vi "AlliGator Phasor Plot Actions.vi"(0 "AlliGator Q Elements in":T6[](array[typedef]), 1 "VI in":refnum<vi>, 2 "Script in":bool, 5 "data value reference in":refnum<data-value>, 7 "AlliGator Q Event in":T7=enum."GUI:Idle", 9 "Data":variant, 11 "error in (no error)":errorcluster, 12 "AlliGator Ctrl Refnums":T8) -> (3 "Script out":bool, 4 "AlliGator Q Elements out":T6[](array[typedef]), 6 "Data Value Reference out":refnum<data-value>, 10 "[Notebook Message]":T1[](array[typedef]) {"Message Style"."Font Size" min=6.0 step=1.0}, 15 "error out":errorcluster)   [LabVIEW 2021, in "AlliGator Action Engine.lvlib"]
doc: "Processes AlliGator phasor plot-related actions."
uses:
  AlliGator Action Engine.lvlib
  Internal Variables/AlliGator Internal Variables v2.ctl
  <vilib>/vision/Image Controls.llb/IMAQ Image.ctl
  Internal Variables/AlliGator Gate Image Set.ctl
  Files/AlliGator FLI Dataset Type.ctl
  Files/AlliGator Data Series Type.ctl
  Dual-Channel Datasets/AlliGator Dataset Channel.ctl
  Settings/AlliGator Gate Arithmetic.ctl
  Source Image/AlliGator Displayed Image.ctl
  Image/Named ROI Description.ctl
  Phasor Graph/AlliGator Decay Metadata v3.ctl
  Decay Analysis/Decay Preprocessing/AlliGator Decay Background Subtraction Info.ctl
  Decay Analysis/Decay Preprocessing/AlliGator Baseline Subtraction Method.ctl
  Graphs/XY Graph/XY Graph Plot Shift Parameters.ctl
  Graphs/XY Graph/XY Graph Plot Shift Method.ctl
  Decay Analysis/Decay Preprocessing/AlliGator Decay Extrapolation Parameters.ctl
  Phasor/Calibration Phasor (m, phi).ctl
  Phasor/Phasor Reference Series.ctl
  Phasor/Phasor Calibration Map v2.ctl
  Phasor/Phasor (g, s).ctl
  Phasor Graph/AlliGator Raw Phasor Plot Data v5.ctl
  Phasor/Phasor Standard Deviation Options.ctl
  Phasor Plot/AlliGator Phasor Multi-Harmonic Data.ctl
  Phasor/Phasor Harmonic Data.ctl
  Decay Fit Parameter Map/AlliGator Decay Fit Options & Parameters v4.ctl
  Fits/IRF(X)PSED/Decay Fit Options v4.ctl
  Fits/Decay Convolution/Decay Model.ctl
  Fits/Residual Type.ctl
  Fits/IRF(X)PSED/Fit Weights Type v2.ctl
  Fits/Non-linear Fitting Method v2.ctl
  Fits/Fit Calculation Method.ctl
  Fits/Non-linear Fitting Algorithm.ctl
  Decay Analysis/Decay Fit/AlliGator Decay Fit Parameter Constraints 2.ctl
  Fits/IRF(X)PSED/Decay Fit Parameters In List.ctl
  Fits/IRF(X)PSED/MLE Baseline Offset Type.ctl
  Decay Analysis/Decay Preprocessing/AlliGator Decay Preprocessing Parameters.ctl
  Fits/IRF(X)PSED/Decay Fit Parameters & Derived Quantities List v2.ctl
  Fits/IRF(X)PSED/Decay Fit Result Constraint.ctl
  Decay Fit Parameter Map/AlliGator Parameter Maps Data.ctl
  AlliGator Q Event.ctl
  GUI/AlliGator Ctrl Refnums.ctl
  GUI/AlliGator Other Ctrl Refnums.ctl
  GUI/AlliGator State Indicator.ctl
  GUI/AlliGator Main Window Tabs.ctl
  GUI/AlliGator Phasor Plot Ctrl Refnums.ctl
  GUI/AlliGator Phasor Graph Ctrl Refnums.ctl
  Phasor/Phasor Calibration Type.ctl
  GUI/AlliGator Dataset Ctrl Refnums.ctl
  GUI/AlliGator Registered Events Ctrl Refnums.ctl
  GUI/AlliGator Image Histogram Control Refnums.ctl
  Histograms/Linear Histogram Options.ctl
  Histograms/Histogram Bin Option.ctl
  Histograms/Histogram Bin Position.ctl
  Decay Fit Parameter Map/AlliGator Decay Fit Map Control Refnums.ctl
  Parameter Map/AlliGator Parameter Map Control Refnums.ctl
  AlliGator Q Element.ctl
  Notebook/Notebook Message Object.ctl
  Rich Text Box/Text Formatting.ctl
  Rich Text Box/Text Colors.ctl
  Rich Text Box/Text Style.ctl
  Rich Text Box/Text Alignment.ctl
  Rich Text Box/Text Format List.ctl
  Globals, Variables, Constants/AlliGator Variables List.ctl
  GUI/AlliGator Image Display Type.ctl
  Palette/Image Palette Information.ctl
  Image/Image Display Palette Type.ctl
  Alligator Elements Order in Action Stack.ctl
  Image/Image Control ROI Description.ctl
  Settings/AlliGator Settings List.ctl
  ROIs/AlliGator ROI Manager Actions.ctl
  Utilities/Read-Write.ctl
  793a9f64-fd61-4161-b52c-76edb5dbf837.vi
  Variant/Variant to Data/Variant to Boolean.vi
  Variant/Variant to Data/Variant to [String].vi
  AlliGator Add Single Action to Stack.vi
  Variant/Variant to Data/Variant to String.vi
  Variant/Variant to Data/Variant to IMAQ Image.vi
  AlliGator Add Action Array to Stack.vi
  ROIs/AlliGator Phasor Plot Image ROI Storage [SGL] v3.vi
  Variant/Variant to Data/Variant to Data.lvlib
  GUI/GUI.lvlib
  Phasor Plot/AlliGator Phasor Plot.lvlib
  Phasor Ratio/AlliGator Phasor Ratio.lvlib
  Phasor Plot Color Map/AlliGator Phasor Plot Color Map.lvlib
  Image/Image.lvlib
  Source Image/AlliGator Source Image.lvlib
  Files/AlliGator Files.lvlib
  Internal Variables/AlliGator Internal Variables.lvlib
  Files/Files.lvlib
  GUI/AlliGator GUI.lvlib
  Globals, Variables, Constants/AlliGator Globals, Variables & Constants.lvlib
  Palette/Palette.lvlib
  ROIs/AlliGator ROIs.lvlib
  Settings/AlliGator Settings.lvlib
  Utilities/Utilities.lvlib
  Sound/Sound.lvlib
  <vilib>/Utility/miscctls.llb/LVPoint32TypeDef.ctl
  Image/Image Control Refnum.ctl
  Image/Image Display Mouse Click Event Data.ctl
  Time/Time.lvlib
  Phasor/Phasor.lvlib
  Notebook/Notebook.lvlib
  Decay Analysis/Decay Preprocessing/AlliGator Decay Preprocessing.lvlib
  Graphs/XY Graph/XY Graph Add-Ons.lvlib
  Phasor Graph/AlliGator Phasor Graph.lvlib
  Fits/Fits.lvlib
  Decay Analysis/Decay Fit/AlliGator Decay Fit.lvlib
  Decay Fit Parameter Map/AlliGator Decay Fit Parameter Map.lvlib
  Rich Text Box/Rich Text Box.lvlib
  Dual-Channel Datasets/AlliGator Dual-Channel Datasets.lvlib
  Histograms/Histogram Window.lvlib
  Parameter Map/AlliGator Parameter Map.lvlib
panel:
  # "see the AlliGator License on the block diagram (Ctrl+E or Window:Show Block Diagram)"
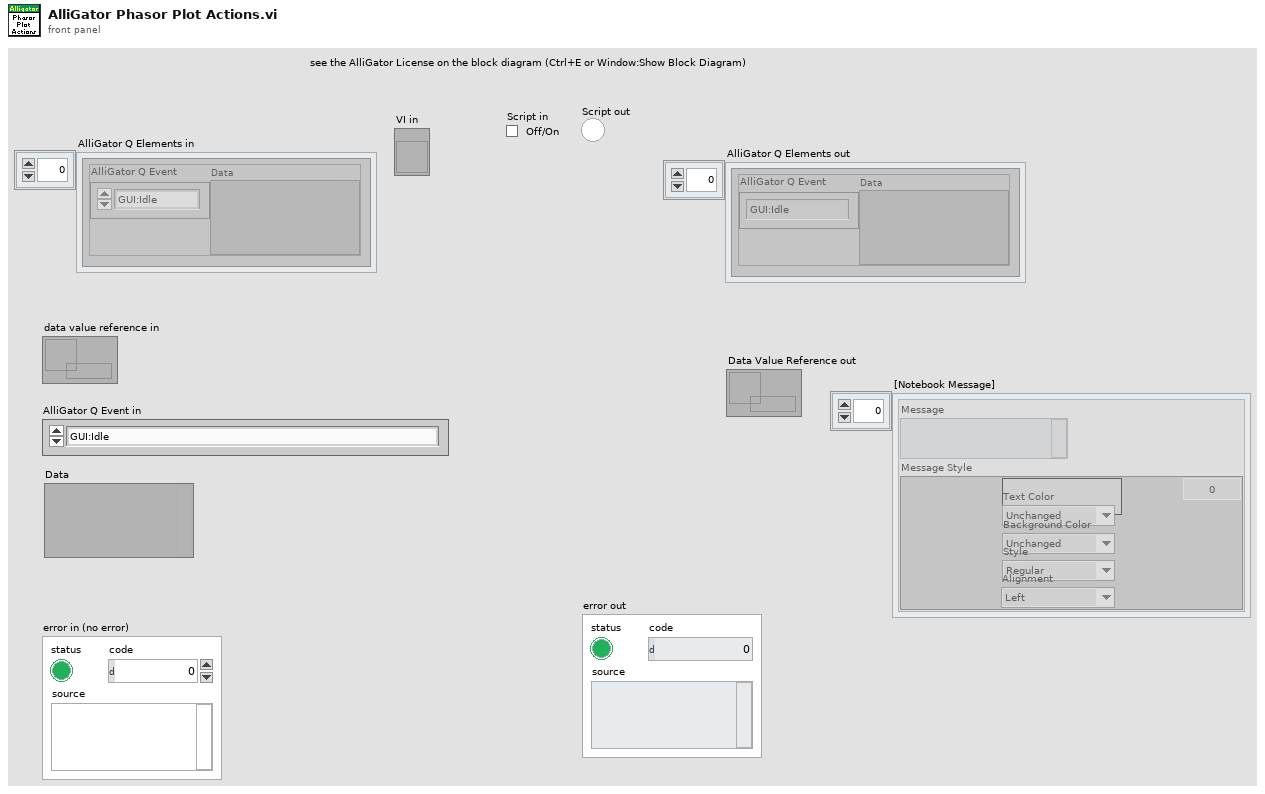
[diagram p1: front panel]
types:
  T1 = typedef "Notebook.lvlib/Notebook Message Object.ctl" = cluster{"Message":string, "Message Style":T2}
  T2 = typedef "Rich Text Box.lvlib/Text Formatting.ctl" = cluster{"Font":string, "Text Color":T3, "Background Color":T3, "Style":T4, "Font Size":dbl, "Alignment":T5}
  T3 = typedef "Rich Text Box.lvlib/Text Colors.ctl" = enum16{"Unchanged", "Black", "Blue", "Cyan", "Maroon", "Gray", "Violet", "Green", "Light Green", "Orange", "Yellow", "Magenta", "Red", "White"}
  T4 = typedef "Rich Text Box.lvlib/Text Style.ctl" = enum16{"Regular", "Bold", "Italic", "Underline", "Strikeout"}
  T5 = typedef "Rich Text Box.lvlib/Text Alignment.ctl" = enum16{"Left", "Right", "Center"}
  T6 = typedef "AlliGator Action Engine.lvlib/AlliGator Q Element.ctl" = cluster{"AlliGator Q Event":T7, "Data":variant}
  T7 = typedef "AlliGator Action Engine.lvlib/AlliGator Q Event.ctl" = enum16{"---- Files ----", "Files:Set Batch Export Files To Save", "Files:Set Dataset Loading & Pre-processing Options", "Files:Check #Frames in Dataset", "Files:Increment Frame Index", "Files:Open Mask Image", "Files:Open White Light Image", "Files:Open Single Dataset", "Files:New Folder of Folders Selected", "Files:Load File (all Types)_Scriptable", "Files:Move Flattened Series to Folders Series", "Files:Select Folder", "Files:Load FLI Dataset", "Files:Load Swiss SPAD 1 Dataset", "Files:Load Swiss SPAD 2 Dataset", "Files:Load .sdt FLI Dataset", "Files:Load .ptu FLI Dataset", "Files:Load .bin FLI Dataset", "Files:Load Single Gate Image Folder", "Files:Load I/m/phi Dataset (deprecated)", "Files:Load Single Image", "Files:Subtract Background File", "Files:Export FLI Dataset", "Files:Load HDF5 FLI Dataset", "Files:Set Destination File Path", "Files:Save Mask Image", "Files:Batch Conversion", "Files:New Folder Selected", "Files:Close FLI Dataset", "Files:Close FLI Dataset Series", "Files:Close White Light Image", "Files:Close Mask Image", "---- FLI Dataset ----", "FLI Dataset:Channel Arithmetic", "FLI Dataset:Export Average Lifetime Map as ASCII", "FLI Dataset:Export User-Defined Quantity Map as ASCII", "FLI Dataset:Python Function FLI Dataset Event", "FLI Dataset:ROI Analysis", "FLI Dataset:Tilted Logistic Square Gated IRF Characteristics Map", "FLI Dataset:Logistic Square Gated IRF Characteristics Map", "FLI Dataset:Square Gated IRF Characteristics Map", "FLI Dataset:Multi-ROI Single-Pixel Phasor Analysis", "FLI Dataset:Multi-ROI Single-Pixel NLSF Analysis", "FLI Dataset:All ROIs IRF Extraction", "FLI Dataset:All ROIs Decay Fit Non-Interactive (Fast + Individual IRF)", "FLI Dataset:All ROIs Phasor Analysis", "FLI Dataset:All ROIs Decay Fit", "FLI Dataset:Fluorescence Decay Statistics", "FLI Dataset:Update Decay Statistics Graph", "FLI Dataset:Get Decay from ROI", "FLI Dataset:All ROIs Average Lifetimes", "FLI Dataset:Save/Load Local IRFs", "FLI Dataset:Clear Local IRFs", "FLI Dataset:Phasor Calibration Maps (# Gates Series) Script", "FLI Dataset:Calibrated Phasor Map Series", "---- FLI Dataset Series ----", "FLI Dataset Series:Sum All Datasets in Series", "FLI Dataset Series:Add Dataset to Accumulated Dataset", "FLI Dataset Series:Display Accumulated Dataset", "FLI Dataset Series:Clear Dataset Series Sum", "FLI Dataset Series:Time-Series Analysis (NLSF)", "FLI Dataset Series:Time-Series Analysis (Phasor)", "---- Image ----", "Image:Update Image Profile Plots", "Image:Image Histogram Cursor Move", "Image:Image Histogram", "Image:Image Contrast", "Image:Set Image Histogram Cursor Move Flag", "Image:Clear Image Overlay", "Image:Use ROI as Search Area", "Image:Set ROI Diameter", "Image:Save Image Data as TIFF", "Image:Save Displayed Image with Overlay", "Image:Save Image Overlay Only", "Image:Save Image as Hot Pixel Mask", "Image:Change Source Image Color Palette", "Image:Copy Image to Clipboard", "Image:Source Image ROI Selection", "Image:Delete All ROIs", "Image:Delete All Unselected ROIs", "Image:Delete ROI", "Image:Merge All ROIs", "Image:Store ROI", "Image:Source Image ROI Storage", "Image:Export ROI Description to Notebook", "Image:Save ROI", "Image:Load ROI", "Image:Paste ROI Definition", "Image:Clear ROI", "Image:Identify ROIs in Mask Image", "Image:Create Complementary ROI", "Image:Create Contour ROI", "Image:Create ROI(s) from Pixels with Peak above Min_Scriptable", "Image:Create ROI(s) from Pixels with Intensity above Min_Scriptable", "Image:Compute ROI Statistics", "Image:Delete ROI(s) based on ROI Characteristics", "Image:Create ROI Grid", "Image:ROI to Individual Pixel ROIs", "Image:Python Function Source Image Event", "Image:Show Phasor Calibration Map ROI Centers", "Image:Convert ROI to Mask Image", "Image:Mouse Move", "Image:Mouse Up", "Image:Set Source Image Mouse Move Flag", "Image:Add Scale Bar Overlay", "Image:Delete Existing ROIs Option", "Image:Overlay ROI Median", "Image:Check Current ROI", "Image:Update True Pixel Value", "---- Decay ----", "Decay:Clear IRF/Reference Plot", "Decay:Add Decay to Graph", "Decay:Smoothen Plot", "Decay:Smoothen Plot Tail", "Decay:Average Selected Plots", "Decay:Extract IRF", "Decay:Optimal IRF Extraction", "Decay:Threshold IRF", "Decay:Fit to Model IRF", "Decay:Fit IRF to Square Gate", "Decay:Fit IRF to Logistic Square Gate", "Decay:Fit IRF to Tilted Logistic Square Gate", "Decay:Create Bounding Cursors Set", "Decay:Export Bounding Cursors Definition to Notebook", "Decay:Denoise Plot", "Decay:Compute Cumulative Function", "Decay:Use as Reference Decay", "Decay:Show Reference Decay/IRF", "Decay:Extrapolate Decay", "Decay:Create Head & Tail Bounding Cursors", "Decay:Store Cursor-defined Head & Tail Fractions", "Decay:Rebin Plot", "Decay:1-Normalize Decay", "Decay:[0-1]-Normalize Plot", "Decay:Straighten Decay", "Decay:Shift Decay", "Decay:Fold Decay", "Decay:Fit Decay", "Decay:Global Fit of Selected Decays", "Decay:Post Global Fit Script", "Decay:Add Global Fit Parameters to Graph", "Decay:Add Decay Parameter(s) to Plot (Graph)", "Decay:Export Decay to Phasor Graph", "Decay:Compute Average Lifetime", "Decay:Plot Convolution", "Decay:Graph Tip Strip Update", "---- Decay Statistics ----", "Decay Statistics:Tip Strip Update", "---- Intensity Time Trace ----", "Intensity Time Trace:Use File Timestamp", "Intensity Time Trace:Load Intensity Corrections File", "Intensity Time Trace:Clear Intensity Corrections File", "Intensity Time Trace:Tip Strip Update", "---- Phasor Plot ----", "Phasor Plot:Build Phasor Plot", "Phasor Plot:Change Phasor Plot Color Palette", "Phasor Plot:Adjust Phasor Plot Display Range", "Phasor Plot:Highlight Image ROI in Phasor Plot", "Phasor Plot:Save Phasor Plot Image with Overlay", "Phasor Plot:Export Complex Phasor Map", "Phasor Plot:Export Phasor Ratio Map", "Phasor Plot:Export Average Lifetime Map", "Phasor Plot:Compute Phase Lifetime Histogram", "Phasor Plot:Compute Phasor Ratio Histogram", "Phasor Plot:Compute Phase Lifetime vs Intensity Scatter Plot", "Phasor Plot:Weber 2-Component Decomposition", "Phasor Plot:Update Phasor Color Map Vertices", "Phasor Plot:Clear Phasor Overlay", "Phasor Plot:Use Segment Extremities as References", "Phasor Plot:Use UC/Segment Intersections as References", "Phasor Plot:Use UC/Principal Axis Intersections as References", "Phasor Plot:Use UC/Linear Fit Intersections as References", "Phasor Plot:Update Phasor Plot Reference", "Phasor Plot:Show Local Phasor Info in Phasor Plot", "Phasor Plot:Update Phasor Plot State", "Phasor Plot:Phasor Plot ROI Storage", "Phasor Plot:Phasor Plot ROI Selection", "Phasor Plot:Python Function Phasor Plot Event", "Phasor Plot:Overlay Phasor ROI, Ratio or Map in Source Image", "Phasor Plot:Compute Decay of Selected Phasors", "Phasor Plot:Phasor at Image Pixel", "Phasor Plot:Mouse Move", "Phasor Plot:Mouse Up", "Phasor Plot:Display Range Mouse Move", "Phasor Plot:Set Mouse Move Flag", "Phasor Plot:Update True Phasor Plot Value", "---- Phasor Graph ----", "Phasor Graph:Get Phasor Value", "Phasor Graph:Create New Phasor Plot Dialog", "Phasor Graph:Update Last Phasor Value", "Phasor Graph:Update Phasor (m, phi)", "Phasor Graph:Remove Single Phasor from Plot", "Phasor Graph:Add Single Phasor to Plot", "Phasor Graph:Remove Phasor Plot", "Phasor Graph:Remove Selected Phasor Plots", "Phasor Graph:Clear Phasor Data", "Phasor Graph:Clear Phasor Graph", "Phasor Graph:Cursor Move", "Phasor Graph:Draw Cursor Connecting Line", "Phasor Graph:Clear Cursor Connecting Line", "Phasor Graph:Find UC Intersection", "Phasor Graph:Use UC/Cursor-Defined Line Intersections", "Phasor Graph:Use Selected Plots Fitted Line/UC Intersections", "Phasor Graph:Use Selected Plots Principal Axis/UC Intersections", "Phasor Graph:Show Single Phasor", "Phasor Graph:Save Single Phasor Plot", "Phasor Graph:Save All Phasor Plots", "Phasor Graph:Load Phasor Plot(s)", "Phasor Graph:Phasor Multiplication", "Phasor Graph:Compute Average Phasor", "Phasor Graph:Compute Multiple Average Phasors (Selected Plots)", "Phasor Graph:Export Single Phasor Plot Phase Lifetimes", "Phasor Graph:Parameter 2 vs Parameter 1 Scatter Plot", "Phasor Graph:Use Cursor n Location", "Phasor Graph:Set Reference n to Current Phase Lifetime Value", "Phasor Graph:Set Reference n to Lifetime Value", "Phasor Graph:Set Cursor n Location", "Phasor Graph:Save Phasor Graph Image", "Phasor Graph:Update SEPL Plot", "Phasor Graph:Export Single Phasor Plot Data", "Phasor Graph:Export Selected Phasor Plots Data", "Phasor Graph:Python Function Phasor Graph Event", "Phasor Graph:Tip Strip Update", "---- Calibration ----", "Calibration:Set Calibration Type", "Calibration:Load/Save Phasor Calibration", "Calibration:Load/Save Phasor Calibration Series", "Calibration:Load/Save Phasor Calibration Map", "Calibration:Use as Calibration", "Calibration:Compute Optimal Calibration from Phasor References", "Calibration:Clear Phasor Calibration", "Calibration:Single Phasor Calibration Information", "Calibration:Use as Calibration Series", "Calibration:Use as Calibration Map", "Calibration:Clear Calibration Series", "Calibration:Phasor Calibration Series Information", "Calibration:Clear Calibration Map", "Calibration:Phasor Calibration Map Information", "Calibration:Apply Phasor Calibration", "Calibration:Update Single Plot Calibration", "Calibration:Update Multiple Plots Calibration", "Calibration:Clear Single Plot Calibration", "Calibration:Clear All Plots Calibrations", "Calibration:Clear Plot(s) Calibration(s)?", "---- Phasor Ratio ----", "Phasor Ratio:Clear Reference n", "Phasor Ratio:Toggle Selected Plot(s)  Lock to Reference 1", "Phasor Ratio:Use as Reference n", "Phasor Ratio:Send Reference n to Notebook", "Phasor Ratio:Toggle Selected Plot(s)  Lock to Reference 2", "Phasor Ratio:Compute Phasor Ratio at Mouse Location", "Phasor Ratio:Compute Phasor Plot's Average Phasor Ratio", "Phasor Ratio:Compute Time-Series Phasor Ratios", "Phasor Ratio:Fit Line to Phasor Ratio Plot", "Phasor Ratio:Save References", "Phasor Ratio:Load References", "Phasor Ratio:Update Phasor Reference 1", "Phasor Ratio:Update Phasor Reference 2", "Phasor Ratio:Move Cursor n to Reference n", "Phasor Ratio:Use as Phasor Reference 1 Lifetime", "Phasor Ratio:Use as Phasor Reference 2 Lifetime", "Phasor Ratio:Export Phasor Ratio Map as ASCII", "Phasor Ratio:Tip Strip Update", "---- Lifetime & Other Parameters Graph ----", "Lifetime:Compute Sliced Mean, SDV and CV Plots", "Lifetime:Plot Decay Shifts", "Lifetime:Plot Histogram", "---- Decay Fit Parameter Map ----", "Decay Fit Parameter Map:Export ROI NLSF Data as ASCII", "Decay Fit Parameter Map:Set Decay Fit Parameter Map Selection", "Decay Fit Parameter Map:Build Decay Fit Parameter Map", "Decay Fit Parameter Map:Change Decay Fit Parameter Map Color Palette", "Decay Fit Parameter Map:Export Decay Fit Parameter Map Data as ASCII", "Decay Fit Parameter Map:Export All Decay Fit Parameter Maps Data as ASCII", "Decay Fit Parameter Map:Selected Parameter Scatterplot", "Decay Fit Parameter Map:Parameter 2 vs Parameter 1 Scatterplot", "Decay Fit Parameter Map:Save Decay Fit Parameter Map Image", "Decay Fit Parameter Map:Save-Load IRFs & Fit Data", "Decay Fit Parameter Map:Update Local Decay Plots", "Decay Fit Parameter Map:Python Function Decay Fit Parameters Map Event", "Decay Fit Parameter Map:Overlay Decay Fit Parameter Map in Source Image", "Decay Fit Parameter Map:Selected Parameter vs Intensity Scatterplot", "Decay Fit Parameter Map:Mouse Up", "Decay Fit Parameter Map:Mouse Move", "Decay Fit Parameter Map:Display Range Mouse Move", "Decay Fit Parameter Map:Change Map Resolution", "Decay Fit Parameter Map:Variance Significance Maps", "Decay Fit Parameter Map:Fit Result Constraints Window", "---- Parameter Map ----", "Parameter Map:Export ROI Parameters Data as ASCII", "Parameter Map:Add Parameter Map Set", "Parameter Map:Delete Parameter Map Set", "Parameter Map:Update Parameter List", "Parameter Map:Build Parameter Map", "Parameter Map:Change Parameter Map Color Palette", "Parameter Map:Export Parameter Map Data as ASCII", "Parameter Map:Export All Parameter Maps Data as ASCII", "Parameter Map:Selected Parameter Scatterplot", "Parameter Map:Parameter 2 vs Parameter 1 Scatterplot", "Parameter Map:Selected Parameter vs Intensity Scatterplot", "Parameter Map:Save Parameter Map Image", "Parameter Map:Save-Load IRFs & Parameter Maps (TODO)", "Parameter Map:Set Parameter Map Selection", "Parameter Map:Python Function Parameter Map Event", "Parameter Map:Overlay Parameter Map in Source Image", "Parameter Map:Update Local Decay Plots", "Parameter Map:Mouse Up", "Parameter Map:Mouse Move", "Parameter Map:Display Range Mouse Move", "---- Generic Graph ----", "Generic Graph:Generic XY Graph Event", "Generic Graph:Python Function XY Graph Event", "Generic Graph:New Plot", "Generic Graph:Save Plot", "Generic Graph:XY Plot Histogram", "Generic Graph:Set XY Graph Plot Name", "Generic Graph:Set Last Cursor Style", "Generic Graph:Tip Strip Update", "---- GUI ----", "GUI:Start Script", "GUI:Type of Displayed Image Changed", "GUI:Gate Image Slide Changed", "GUI:Show Busy Icon", "GUI:Show Busy Icon & Abort Button", "GUI:Hide Busy Icon", "GUI:Hide Busy Icon & Abort Button", "GUI:Abort", "GUI:End Script", "GUI:Start Timing", "GUI:End Timing", "GUI:Set State Indicator", "GUI:Send Parameters JSON Strings to Clipboard", "GUI:Set Gate Step", "GUI:Idle", "GUI:Initialization", "GUI:Quit", "GUI:Increment Dataset Index", "GUI:Set Dataset Index to -1", "GUI:Time Series Slider Moved", "GUI:Time Series Slider Changed", "GUI:Toggle Playback or Loop", "GUI:Playback Script", "GUI:Set Phasor Frequency", "GUI:Open Window", "GUI:Start Test Script", "GUI:End Test Script", "GUI:Set Verbose Mode", "GUI:Set Verbose Settings Mode", "DEBUG"}
  T8 = typedef "AlliGator GUI.lvlib/AlliGator Ctrl Refnums.ctl" = cluster{"Other AlliGator Ctrl Refnums":T9, "Phasor Plot Ctrl Refnums":T10, "Phasor Graph Ctrl Refnums":T11, "Dataset Control Refnums":T12, "Registered Events Ctrl Refnums":T13, "Image Histogram Ctrl Refnums":T14, "Decay Fit Map Ctrl Refnums":T15, "Parameter Map Ctrl Refnums":T16}
  T9 = typedef "AlliGator GUI.lvlib/AlliGator Other Ctrl Refnums.ctl" = cluster{"State Indicators":refnum<vi>, " Progress Bar":refnum<vi>, "Decay Graph Active":refnum<vi>, "Decay Statistics Bin":refnum<vi>, "Time Step":refnum<vi>, "Use File Timestamp":refnum<vi>, "Tab Control":refnum<vi>, "CPU":refnum<vi>, "Abort Fit":refnum<vi>, "Dataset File/Folder Path":refnum<vi>, "Abort ROI Creation":refnum<vi>, "Event LED":refnum<vi>, "Dataset File/Folder Path 2":refnum<vi>, "Dataset File/Folder Path 3":refnum<vi>, "Dataset File/Folder Path 4":refnum<vi>, "Dataset File/Folder Path 5":refnum<vi>, "Dataset File/Folder Path 6":refnum<vi>, "Dataset File/Folder Path 7":refnum<vi>, "Dataset File/Folder Path 8":refnum<vi>, "Dataset File/Folder Path 9":refnum<vi>, "Dataset File/Folder Path 10":refnum<vi>, "Dataset File/Folder Path 11":refnum<vi>}
  T10 = typedef "AlliGator GUI.lvlib/AlliGator Phasor Plot Ctrl Refnums.ctl" = cluster{"Phasor Ratio":refnum<vi>, "Modulus Lifetime":refnum<vi>, "Phasor at cursor (m, phi)":refnum<vi>, "Phase Lifetime":refnum<vi>, "Phasor at cursor (g, s)":refnum<vi>, "Phasor Plor Average Lifetime":refnum<vi>, "Phasor Plot Active":refnum<vi>, "Save Phasor Plot":refnum<vi>, "Image Overlay Color":refnum<vi>, "Phasor Plot Color Scale":refnum<vi>, "Reference 1 Button":refnum<vi>, "Reference 2 Button":refnum<vi>, "True Phasor Plot Value":refnum<vi>}
  T11 = typedef "AlliGator GUI.lvlib/AlliGator Phasor Graph Ctrl Refnums.ctl" = cluster{"Phasor Ratio":refnum<vi>, "Modulus Lifetime":refnum<vi>, "Phasor at cursor (m, phi)":refnum<vi>, "Phase Lifetime":refnum<vi>, "Phasor at cursor (g, s)":refnum<vi>, "Phasor Graph Average Lifetime":refnum<vi>, "Phasor Graph Active":refnum<vi>, "Save Phasor Graph":refnum<vi>, "Phasor Frame Slide":refnum<vi>, "Single Step Phasor":refnum<vi>, "Calibration Type":refnum<vi>, "Show Line":refnum<vi>, "Phase Lifetime 1":refnum<vi>, "Phase Lifetime 2":refnum<vi>, "Phasor Graph Frequency":refnum<vi>, "Phasor Reference 1 Control":refnum<vi>, "Phasor Reference 2 Control":refnum<vi>, "Calibration Lifetime":refnum<vi>, "Phase Lifetime SDV":refnum<vi>, "Average Lifetime SDV":refnum<vi>, "Phasor Ratio SDV":refnum<vi>, "Modulus Lifetime SDV":refnum<vi>}
  T12 = typedef "AlliGator GUI.lvlib/AlliGator Dataset Ctrl Refnums.ctl" = cluster{"Current Data":refnum<vi>, "Gate Image Slide":refnum<vi>, "Time Point Slide":refnum<vi>, "Current Time Stamp":refnum<vi>, "Save Image":refnum<vi>, "Displayed Image":refnum<vi>, "Overlay Mode":refnum<vi>, "Phasor Overlay Color":refnum<vi>, "Image Color Scale":refnum<vi>, "Use ROI as Search Area":refnum<vi>, "Source Image ROI Color":refnum<vi>, "True Pixel Value":refnum<vi>}
  T13 = typedef "AlliGator GUI.lvlib/AlliGator Registered Events Ctrl Refnums.ctl" = cluster{"Time Point Slider":refnum<vi>, "Phasor Plot Display Range":refnum<vi>, "Decay Graph":refnum<vi>, "Decay Statistics Graph":refnum<vi>, "Intensity Time Trace":refnum<vi>, "Phasor Graph":refnum<vi>, "Phasor Ratio Graph":refnum<vi>, "Lifetime Graph":refnum<vi>, "Phasor Plot Display":refnum<vi>, "Source Image Display":refnum<vi>, "Decay Fit Parameter Map Display Range":refnum<vi>, "Decay Fit Parameter Map Display":refnum<vi>, "Parameter Map Display Range":refnum<vi>, "Parameter Map Display":refnum<vi>, "Phasor Plot Display Range":refnum<vi>}
  T14 = typedef "AlliGator GUI.lvlib/AlliGator Image Histogram Control Refnums.ctl" = cluster{"Image Histogram":refnum<vi>, "Image Histogram Options":refnum<vi>, "Image Histogram Active":refnum<vi>, "Image Histogram Upper Percentile":refnum<vi>, "Image Histogram Lower Percentile":refnum<vi>, "Auto-Adjust Contrast":refnum<vi>}
  T15 = typedef "AlliGator Decay Fit Parameter Map.lvlib/AlliGator Decay Fit Map Control Refnums.ctl" = cluster{"Decay Fit Parameter Map Color Scale":refnum<vi>, "Decay Fit Parameter":refnum<vi>, "Max Parameter":refnum<vi>, "Min Parameter":refnum<vi>, "Decay Fit Parameter Map Display":refnum<vi>, "Decay Fit Parameter Map Display Range":refnum<vi>, "Decay Parameter Map X":refnum<vi>, "Decay Parameter Map Y":refnum<vi>, "Decay Parameter Map Value":refnum<vi>}
  T16 = typedef "AlliGator Parameter Map.lvlib/AlliGator Parameter Map Control Refnums.ctl" = cluster{"Parameter Map Color Scale":refnum<vi>, "Map Parameter":refnum<vi>, "Max Parameter":refnum<vi>, "Min Parameter":refnum<vi>, "Parameter Map Display":refnum<vi>, "Parameter Map Display Range":refnum<vi>, "Parameter Map Set":refnum<vi>, "Parameter Map X":refnum<vi>, "Parameter Map Y":refnum<vi>, "Parameter Map Value":refnum<vi>}
  T17 = typedef "Notebook.lvlib/Text Format List.ctl" = enum16{"Message", "Result", "Error", "Setting", "Verbose", "Warning"}
  T18 = typedef "AlliGator Action Engine.lvlib/Alligator Elements Order in Action Stack.ctl" = enum16{"Enqueue 2 AFTER 1", "Enqueue 2 BEFORE 1"}
  T19 = typedef "AlliGator GUI.lvlib/AlliGator Image Display Type.ctl" = enum16{"Source Image", "Phasor Plot", "Decay Fit Parameter Map", "Parameter Map"}
  T20 = typedef "AlliGator Globals, Variables & Constants.lvlib/AlliGator Variables List.ctl" = enum16{"---- GUI ----", "GUI:Initialization Status", "GUI:State Indicators Refnum", "GUI:Original AlliGator Menu Items", "GUI:Current Action Loop State", "GUI:Script in progress", "GUI:Playback", "GUI:Loop Playback", "GUI:Search ROI Used", "GUI:Search ROI", "Decay Graph Max Legend Size", "Intensity Graph Max Legend Size", "Decay Statistics Graph Max Legend Size", "Phasor Graph Max Legend Size", "Phasor Ratio Graph Max Legend Size", "Lifetime Graph Max Legend Size", "---- Files ----", "Files:Export Dataset Frames as Individual Files", "Files:Show Batch Export Help Balloons", "Files:Frames in Dataset", "Files:ptu File Frame Start Indices", "Files:Current Frame in Dataset", "Files:Current Frame Timestamp", "Files:Dataset Loaded", "Files:Dataset Metadata", "Files:Dataset Channel", "Files:Dataset Data Description", "Files:Background Dataset Metadata", "Files:Background Dataset Channel", "Files:Background Dataset Data Description", "Files:Background File Subtraction", "Files:Background File Path", "Files:Background File Pile-up Correction", "Files:Background File Pixel Well Capacity", "Files:Background File Scaling Factor", "Files:Current Dataset Load Settings", "Files:Dataset Path", "Files:ICCD-specific Information", "Files:Macrotime Gate Separation", "------ Python Plugins ------", "Python Plugins:Information", "Python Plugins:Python Session", "Python Plugins:Valid Python Session?", "---- Source Image ----", "Source Image:ROIs", "Source Image:Current ROI", "Source Image:ROI Event Refnum", "X_Source Image:Display Range", "X_Source Image:Palette Information", "X_Source Image:Type of Displayed Image", "X_Time Gate Slider", "Source Image:Palette List", "Source Image:Scale", "Source Image:ROI Overlay Color", "Source Image:Overlay to Erase", "Source Image:Is Displayed Image Accumulated", "Source Image:White Light Image Modified", "Source Image:Mask Image Modified", "---- Image Profile Window ----", "Image Profile:Window Event Refnum", "Image Profile:IntensityType", "Image Profile:Intensity Average Type", "Image Profile:Intensity-weighted SDV", "Image Profile:Box Profile Type", "Image Profile:Window Open", "Image Profile:Plotted Fit Parameter", "------ Phasor Graph -------", "Phasor Graph:Show Line", "---- Phasor Plot ---", "Phasor Plot:Parameters Changed", "Phasor Plot:FLI Dataset Modified since last Calculation", "Phasor Harmonics Data", "Selected Phasor Harmonics", "Phasor Harmonic Manager Event Refnum", "Phasor Plot:ROIs", "Phasor Plot:Current ROI", "Phasor Plot:ROI Event Refnum", "Phasor Plot:Image Reference Points", "Phasor Plot:Computed", "Phasor Plot:Palette Information", "Phasor Plot:Palette List", "Phasor Plot:Phasor Ratio Palette Information", "Phasor Plot:Phasor Ratio Palette List", "Phasor Plot:Image Scale", "Phasor Plot:Image Overlay to Erase", "Phasor Plot:Image Elements to Update", "Phasor Plot:Current Calculation Parameters", "Phasor Plot:Current Calibration Options", "Phasor Plot:Reset Cumulated Phasor Plot", "Phasor Plot:Reference 1", "Phasor Plot:Lifetime Reference 1", "Phasor Plot:Reference 1 Frequency", "Phasor Plot:Reference 2", "Phasor Plot:Lifetime Reference 2", "Phasor Plot:Reference 2 Frequency", "---- Decay Analysis ----", "Number of Selected Decays to Fit", "LS Fit Results", "LAR Fit Results", "BS Fit Results", "Last Decay Max - Min", "Best Fit Parameters", "Best Fit Parameter Names", "Actual Size X", "Actual Size Y", "Binning X", "Binning Y", "Actual # Gates", "Dataset Number", "Gates to...", "Gates Skipped", "Gates to keep", "Gate Step", "Gate Separation", "Reversed Gates", "Pile-up Correction", "Pixel Well Capacity", "Background Subtracted", "Background Subtraction Method", "Background Definition Range", "Background File (deprecated)", "Number of Dataset Accumulated", "Array of Accumulated Dataset Paths", "Do Averaged Datasets", "Destination File Path", "Process Plot Target", "Use 1/D as Phasor Frequency", "---- Decay Fit Parameter Map -----", "Decay Fit Parameter Map:Palette Information", "Decay Fit Parameter Map:Palette List", "Decay Fit Parameter Map:X Resolution", "Decay Fit Parameter Map:Y Resolution", "Decay Fit Parameter Map:Use Decay Fit Result Constraints", "Decay Fit Parameter Map:Decay Fit Result Constraints", "Decay Fit Parameter Map:Decay Fit Result Constraints Applied", "---- Parameter Map ----", "Parameter Map:Palette Information", "Parameter Map:Palette List", "------- Local Decay Window ---------", "Local Decay Graph Window:Event Refnum", "Local Decay Graph Window:Use normalized IRF for convolution", "----- Miscellaneous ----", "Misc:Skippable Dialog Windows Status"}
  T21 = typedef "Palette.lvlib/Image Palette Information.ctl" = cluster{"Palette Name [# Colors,int?,inv?]":string, "Palette Type":T22, "Palette Colors":u32[], "Interpolate?":bool}
  T22 = typedef "Image.lvlib/Image Display Palette Type.ctl" = u32
  T23 = typedef "AlliGator Settings.lvlib/AlliGator Settings List.ctl" = enum16{"GUI:Visible Settings Tab", "GUI:Last Run Version", "Source Image:Use Image Histogram for Contrast", "Source Image:Low Count Pixels Rejection Options", "Source Image:High Count Pixels Rejection Options", "Source Image:Use Image Brightness", "Source Image:Blend Overlay with Image Background", "Source Image:Use Fixed ROI Diameter", "Source Image:ROI Diameter", "Source Image:ROI Center Color", "Source Image:Peak Threshold", "Source Image:Intensity Threshold", "Source Image:Image Binning Options", "Source Image:Image Smoothing Options", "Source Image:Image Histogram Active", "Source Image:Invert Binary Mask", "Source Image:Hot Pixel Removal", "Source Image:Overlay Analyzed ROI Center", "Source Image:Auto-Adjust Contrast", "Source Image:Histogram Lower Percentile", "Source Image:Histogram Upper Percentile", "Source Image:Save Source Image", "Source Image:Scale Bar Options", "Source Image:Image Resolution (Pixel Size)", "Source Image:Flatfield Correction", "Source Image:Show Dead Left Columns Correction", "Source Image:Dead Left Columns Correction", "Source Image:Image Pre-Processing Operations Order", "Source Image:Overlay ROI Median", "Source Image:Median Overlay Color", "Data Information:Gate Width", "Data Information:Nanotime Gate Separation", "Data Information:Macrotime Gate Separation", "Data Information:Gate Step", "Data Information:# Gates", "Data Information:Gate Image Exposure", "Data Information:Gate Image Integration", "Data Information:Gates to Skip", "Data Information:Gates to Keep", "Data Information:Define Gates to", "Data Information:Channel Name", "Data Information:Available Channel Names", "Data Information:Channel Arithmetic", "Data Information:Background File Subtraction", "Data Information:Background File", "Data Information:Background Scaling Factor", "Data Information:Background Pile-up Correction", "Data Information:Background Pixel Well Capacity", "Data Information:Laser Period", "Data Information:SYNC Period", "Data Information:Pile-up Correction", "Data Information:Pixel Well Capacity", "Data Information:Dataset Scaling Factor", "Fluorescence Decay_Decay Pre-Processing:Reverse Gates", "Fluorescence Decay_Decay Pre-Processing:Verbose Decay Pre-Processing", "Fluorescence Decay_Decay Pre-Processing:Use Decay Pre-Processing", "Fluorescence Decay_Decay Pre-Processing:Background Subtraction", "Fluorescence Decay_Decay Pre-Processing:Background Definition Range", "Fluorescence Decay_Decay Pre-Processing:Baseline Subtraction Method", "Fluorescence Decay_Decay Pre-Processing:Decay Pre-Processing Operations Order", "Fluorescence Decay_Decay Pre-Processing:Smoothing Parameter", "Fluorescence Decay_Decay Pre-Processing:Shift Decay", "Fluorescence Decay_Decay Pre-Processing:Decay Shift Parameters", "Fluorescence Decay_Decay Pre-Processing:Fold Decay", "Fluorescence Decay_Decay Pre-Processing:# Folds", "Fluorescence Decay_Decay Pre-Processing:1-Normalize Decay", "Fluorescence Decay_Decay Pre-Processing:[0-1]-Normalize Decay", "Fluorescence Decay_Decay Pre-Processing:Smoothen Decay", "Fluorescence Decay_Decay Pre-Processing:Extrapolate Decay", "Fluorescence Decay_Decay Pre-Processing:Use Periodicity", "Fluorescence Decay_Decay Pre-Processing:Use Cursors", "Fluorescence Decay_Decay Pre-Processing:Tail Fraction", "Fluorescence Decay_Decay Pre-Processing:Head Fraction", "Fluorescence Decay_Decay Pre-Processing:Additional Points", "Fluorescence Decay_Decay Pre-Processing:Straighten Decay", "Fluorescence Decay_Decay Pre-Processing:Constant Background", "Fluorescence Decay_Decay Pre-Processing:Pixel-Normalize Decay", "Fluorescence Decay_Advanced Analysis:Extract IRF instead of Decay", "Fluorescence Decay_Advanced Analysis:IRF Extraction Options", "Fluorescence Decay_Advanced Analysis:IRF Optimization Options", "Fluorescence Decay_Advanced Analysis:Square Pulse Options", "Fluorescence Decay_Advanced Analysis:IRF Order", "Fluorescence Decay_Advanced Analysis:IRF Time Constants", "Fluorescence Decay_Advanced Analysis:Wavelet Analysis Options", "Fluorescence Decay_Advanced Analysis:Average Lifetime Options", "Fluorescence Decay_Fit Options:Fit Options", "Fluorescence Decay_Fit Options:Use Legacy Fitting Approach", "Fluorescence Decay_Fit Options:Use Data Information Laser Period", "Fluorescence Decay_Fit Parameters:Displayed Fit Parameters", "Fluorescence Decay_Fit Parameters:Fit Parameter Constraints", "Fluorescence Decay_Fit Parameters:Export Tabulated Results", "Fluorescence Decay_Fit Parameters:MLE Baseline Offset Type", "Fluorescence Decay_Fit Parameters:MLE Baseline Offset", "Fluorescence Decay_Fit Parameters:Guess Parameter Names", "Fluorescence Decay_Fit Parameters:Guess Parameter Values", "Fluorescence Decay_Fit Parameters:Guess Parameters Options", "Fluorescence Decay_Fit Parameters:Optimal Offset Selection Criterion", "Fluorescence Decay_Styles:Show Last Decay Only", "Fluorescence Decay_Styles:Decay Graph Color Array", "Fluorescence Decay:Decay Graph Active", "Fluorescence Decay Statistics:Min Peak Value", "Fluorescence Decay Statistics:Reject Low Decay Peak Pixels", "Fluorescence Decay Statistics:Reject High Decay Peak Pixels", "Fluorescence Decay Statistics:Max Peak Value", "Time Traces:Use File Timestamp", "Time Traces:Time Step", "Time Traces:Use Intensity Correction File", "Time Traces:Intensity Correction File", "Phasor Plot:Phasor Plot Smoothing Options", "Phasor Plot:Phasor Plot Size", "Phasor Plot:Phasor Plot Graphics Options", "Phasor Plot:Cumulative Phasor Plot", "Phasor Plot:Use Phasor Brightness", "Phasor Plot:Blend Overlay with Phasor Background", "Phasor Plot:Save Phasor Plot", "Phasor Plot:Show References", "Phasor Plot:Phasor Ratio Decay Range", "Phasor Plot:Exponential Fading", "Phasor Plot:Phasor Ratio Reference Colors", "Phasor Plot:Reference Radius", "Phasor Plot:Show Color Map Vertices", "Phasor Plot:Phasor Plot Active", "Phasor Plot:Phasor Ratio Color Map Type", "Phasor Plot:Phasor Ratio Color Map", "Phasor Plot:Phasor Ratio Display Range", "Phasor Plot:Selected Image ROI(s)", "Phasor Plot:All Image ROIs", "Phasor Plot:Selected Phasor Plot ROI(s)", "Phasor Plot:All Phasor Plot ROIs", "Phasor Plot:Phasor Ratio Color-Coded Quantity", "Phasor Plot:Store Phasor Harmonics", "Phasor Plot:Draw Reference Segment", "Phasor Plot:User-Defined Quantity", "Phasor Plot:Color Scale High Color", "Phasor Plot:Color Scale Low Color", "Phasor Plot:Intensity-weighted Phasor Plot", "Phasor Graph:Phasor Frequency", "Phasor Graph:Phasor Ratio Type", "Phasor Graph:Pixel-level Phasor Computation", "Phasor Graph:Save Phasor Graph", "Phasor Graph:Phasor Graph Active", "Phasor Graph:Phasor SDV Options", "Phasor Graph:Intensity-weighted Phasor Graph", "Phasor Graph:Define Shortest Lifetime as", "Phasor Calibration:Use Backup Calibration if needed", "Phasor Calibration:Backup Calibration Type", "Phasor Calibration:Calibration Type", "Phasor Calibration:Calibration Lifetime", "Phasor Calibration:Calibration Map Algorithm", "Single-Exponential Phasor Locus (SEPL):Gate Parameters", "Single-Exponential Phasor Locus (SEPL):User-defined Gate", "Single-Exponential Phasor Locus (SEPL):User-defined IRF", "Single-Exponential Phasor Locus (SEPL):Phasor Parameters", "Single-Exponential Phasor Locus (SEPL):Decay & IRF Parameters", "Single-Exponential Phasor Locus (SEPL):Display Parameters", "Lifetime Analysis:Decay Analysis Parameters", "Lifetime Analysis:Lifetime Map Active", "Plugins:Python Settings", "Miscellaneous:Verbose Mode", "Miscellaneous:Beep after Script", "Miscellaneous:Saved Image File Format", "Miscellaneous:Exported Gate Image Settings", "Miscellaneous:Include Loading in Timing", "Miscellaneous:Verbose Settings Mode", "Miscellaneous:Histogram Options", "Miscellaneous:Beep on Error", "Miscellaneous:# Logical Processors Used", "Miscellaneous:ROI Description Max Characters", "Miscellaneous:Verbose Error Mode", "Miscellaneous:Transparent Mask Color"}
  T24 = typedef "Image.lvlib/Image Control ROI Description.ctl" = cluster{"Image Control Label":string, "ROI Descriptor":T25}
  T25 = typedef "ROI Descriptor" = cluster{"Global Rectangle":i32[], "Contours":cluster{"ID":enum32{"External", "Internal"}, "Type":u32, "Coordinates":i32[]}[]}
  T26 = typedef "Image.lvlib/Image Display Mouse Click Event Data.ctl" = cluster{"Image Control Refnum":T27, "Mouse Coordinates":T28}
  T27 = typedef "Image.lvlib/Image Control Refnum.ctl" = refnum<vi>
  T28 = typedef "LVPoint32TypeDef.ctl" = cluster{"Horizontal":i32, "Vertical":i32}
  T29 = typedef "AlliGator ROIs.lvlib/AlliGator ROI Manager Actions.ctl" = enum16{"Undefined", "Delete Current ROI", "Delete All Unselected ROIs", "Delete Multiple ROIs", "Delete All ROIs", "Swap ROIs", "Insert ROI", "Update Current ROI Descriptor", "Rename Current ROI", "Store New ROI", "Store Multiple ROIs", "Select Next ROI", "Select Previous ROI", "Find Selected ROI", "Show All ROIs", "Update ROI Manager Window", "Merge All ROIs", "Unmerge ROI", "Set Selected ROI by ID"}
  T30 = typedef "Utilities.lvlib/Read-Write.ctl" = enum16{"Read", "Write"}
  T31 = typedef "Phasor.lvlib/Phasor (g, s).ctl" = cluster{"g":dbl, "s":dbl}
  T32 = typedef "AlliGator GUI.lvlib/AlliGator State Indicator.ctl" = cluster{"Phasor Calibration Defined":bool, "Phasor Calibration Series Defined":bool, "Phasor Calibration Map Defined":bool, "Phasor Ratio Reference 1 Defined":bool, "Phasor Ratio Reference 2 Defined":bool, "Phasor Ratio Lifetime Reference 1 Defined ":bool, "Phasor Ratio Lifetime Reference 2 Defined":bool, "Phasor Calibration Used":bool, "Phasor Calibration Series Used":bool, "Phasor Calibration Map Used":bool, "Dataset Update Needed":bool, "Phasor Plot Update Needed":bool, "Reference/IRF Defined":bool, "Individual IRFs Defined":bool}
  T33 = typedef "Image.lvlib/Image Display User Event Data.ctl" = cluster{"Image Control Refnum":T27, "Coords":T28, "button info":cluster{"button 1":bool, "button 2":bool, "button 3":bool, "button 4":bool}, "keys pressed":enum16{"0", "1", "2", "3", "4", "5", "6", "7", "8", "9", "A", "B", "C", "D", "E", "F", "G", "H", "I", "J", "K", "L", "M", "N", "O", "P", "Q", "R", "S", "T", "U", "V", "W", "X", "Y", "Z", "F1", "F2", "F3", "F4", "F5", "F6", "F7", "F8", "F9", "F10", "F11", "F12", "F13", "F14", "F15", "ADD", "BACK", "BACKSLASH", "CAPITAL", "COMMA", "DECIMAL", "DELETE", "DIVIDE", "DOWN", "END", "EQUALS", "ESCAPE", "GRAVE (`)", "HOME", "INSERT", "LBRACKET", "LCONTROL", "LEFT", "L ALT", "LSHIFT", "LWIN", "MINUS", "MULTIPLY", "NEXT", "NUMLOCK", "NUMPAD_0", "NUMPAD_1", "NUMPAD_2", "NUMPAD_3", "NUMPAD_4", "NUMPAD_5", "NUMPAD_6", "NUMPAD_7", "NUMPAD_8", "NUMPAD_9", "PAUSE", "PERIOD", "PRIOR (PG UP)", "RBRACKET", "RCONTROL", "RETURN", "RIGHT", "R ALT", "RSHIFT", "RWIN", "SCROLL", "SEMICOLON", "SLASH", "SPACE", "SUBTRACT", "TAB", "UP", "ENTER (num pad)", "' (quote)"}[]}
  T34 = typedef "AlliGator GUI.lvlib/AlliGator Image Mouse Up Event Data.ctl" = cluster{"Current ROI Tool":u32, "ROI Descriptor":T35, "Shift":bool, "Alt":bool, "Image Display Refnum":T27}
  T35 = typedef "Image.lvlib/Image ROI Descriptor.ctl" = cluster{"Global Rectangle":i32[], "Contours":T36[]}
  T36 = typedef "Image.lvlib/Image Contour Definition.ctl" = cluster{"Contour Type":T37, "ROI Type":T38, "Points":i32[]}
  T37 = typedef "Image.lvlib/Image Contour ID.ctl" = enum32{"External", "Internal"}
  T38 = typedef "Image.lvlib/Image ROI Type.ctl" = enum16{"No Selection", "Point", "Line", "Rectangle", "Oval", "Polygon", "Freehand Region", "Annulus", "Unused2", "Unused3", "Broken Line", "Freehand Line", "Rotated Rectangle"}
  T39 = typedef "Image.lvlib/Image Color Scale Information.ctl" = cluster{"Scale.Maximum":dbl, "Scale.Minimum":dbl, "Scale.High Color":u32, "Scale.Low Color":u32}
  T40 = typedef "IMAQ Image.ctl" = refnum<image>
  T41 = cluster{"Global Rectangle":i32[], "Contours":cluster{"Contour Type":u32, "ROI Type":u32, "Points":i32[]}[]}
  T42 = typedef "Image.lvlib/Image Save File Format.ctl" = enum16{"PNG", "JPEG", "BMP"}
  T43 = typedef "Image.lvlib/Image Point.ctl" = cluster{"X":i32, "Y":i32}
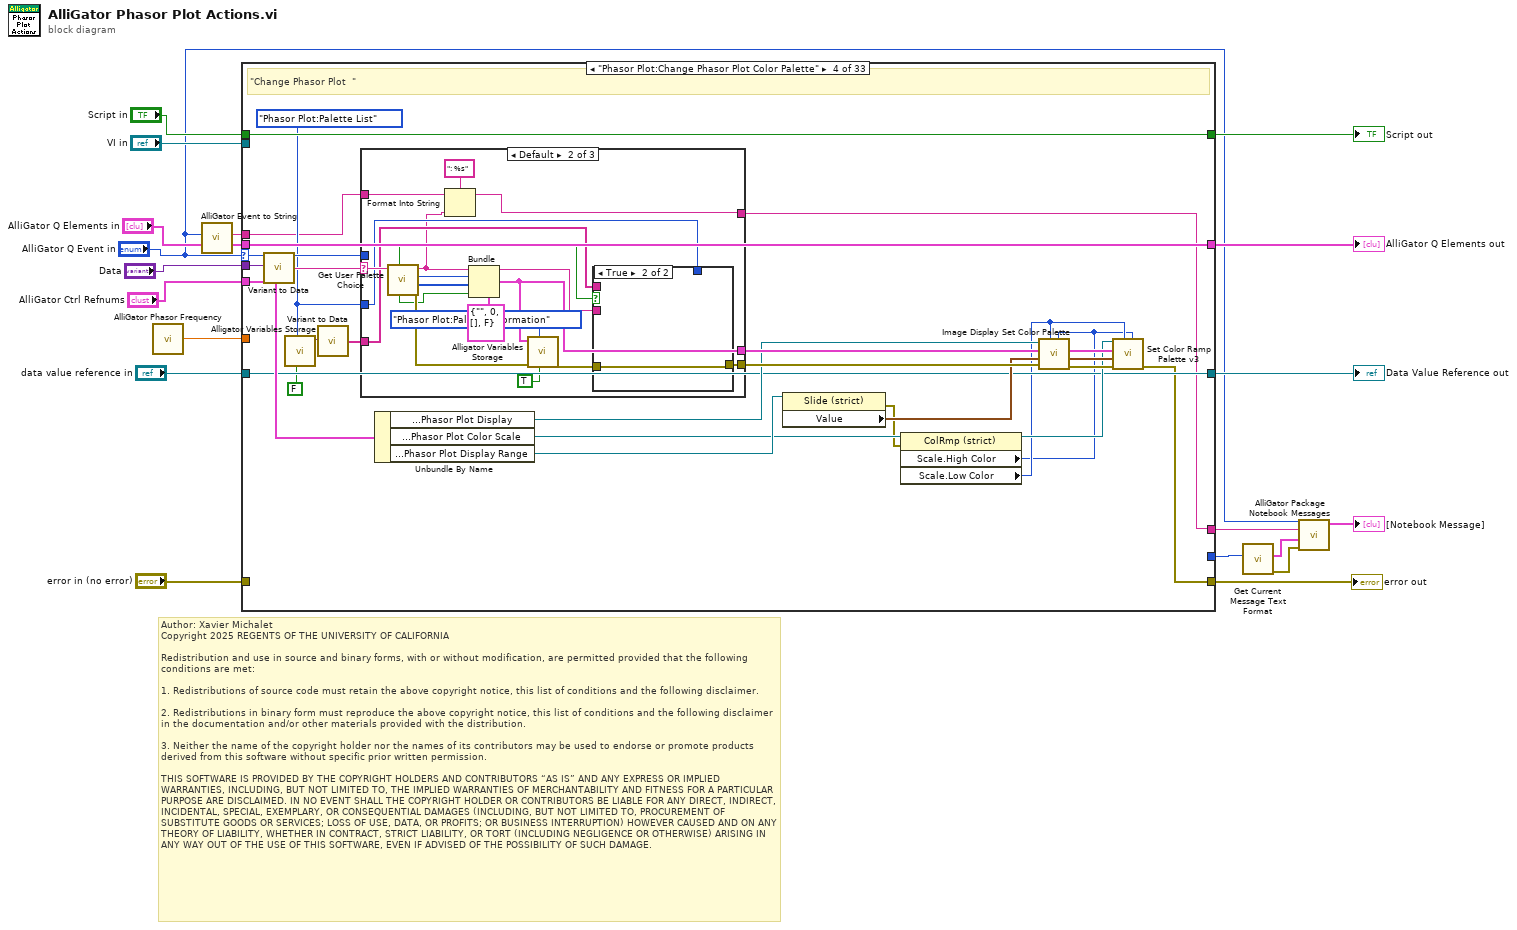
[diagram p0: block diagram]
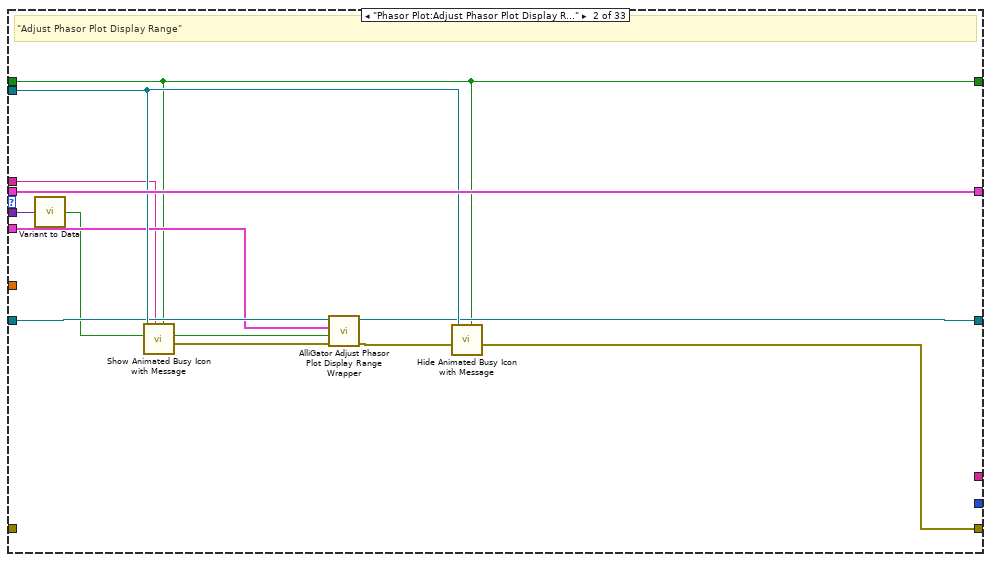
[diagram p3: hidden frame]
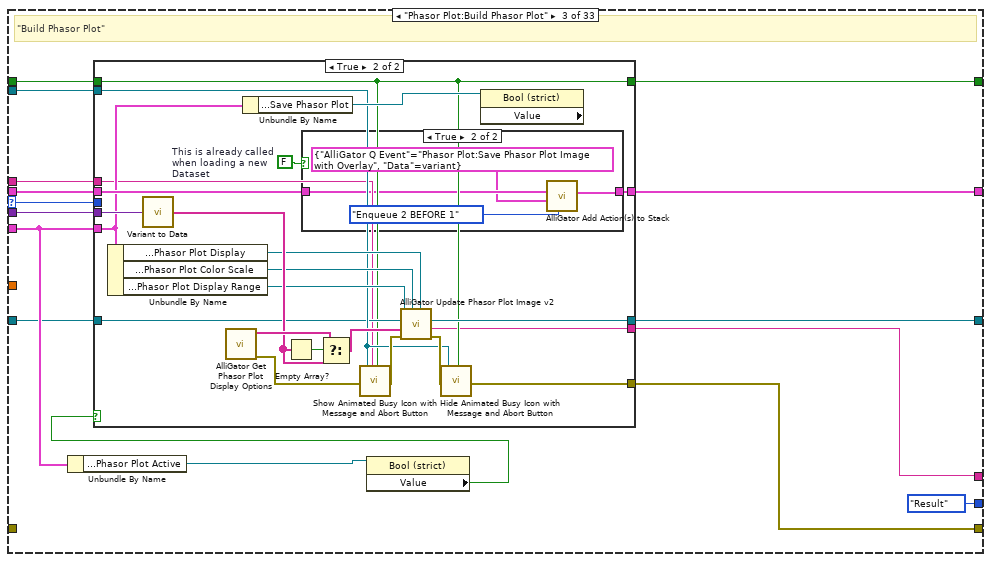
[diagram p4: hidden frame]
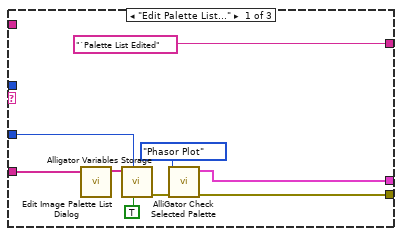
[diagram p7: hidden frame]
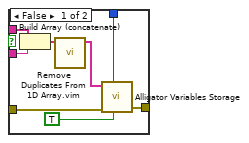
[diagram p8: hidden frame]
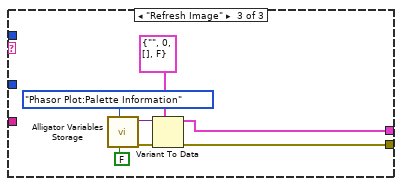
[diagram p9: hidden frame]
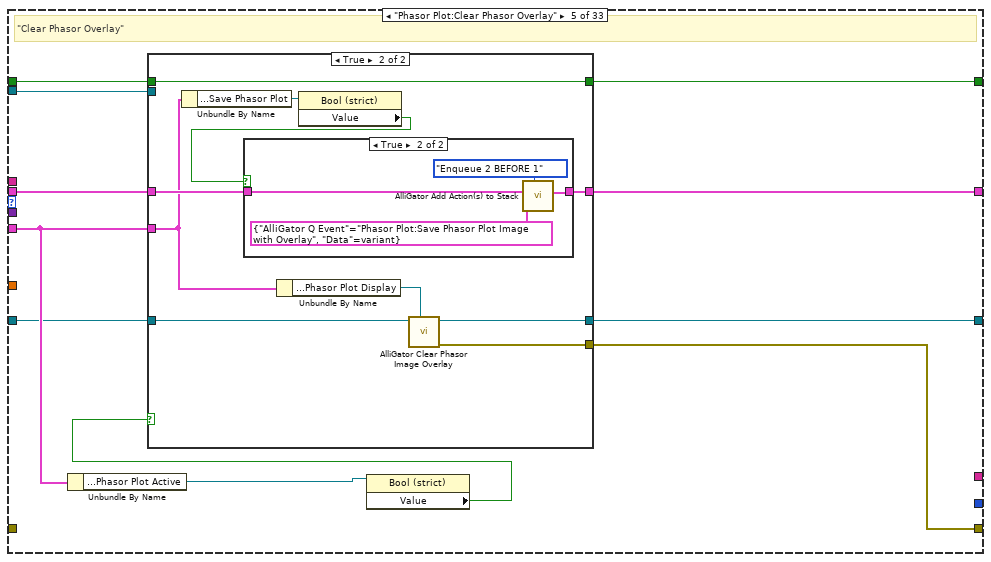
[diagram p10: hidden frame]
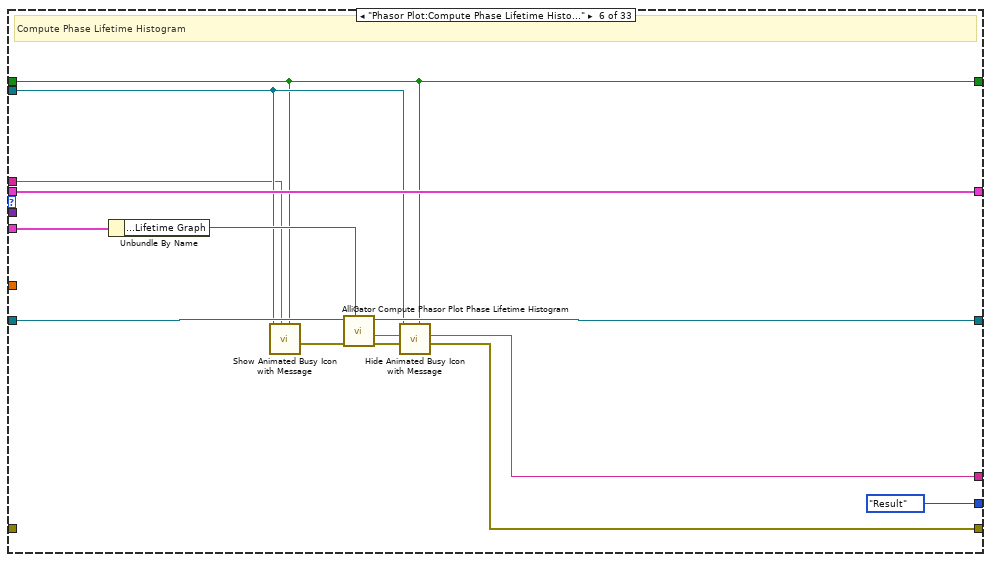
[diagram p13: hidden frame]
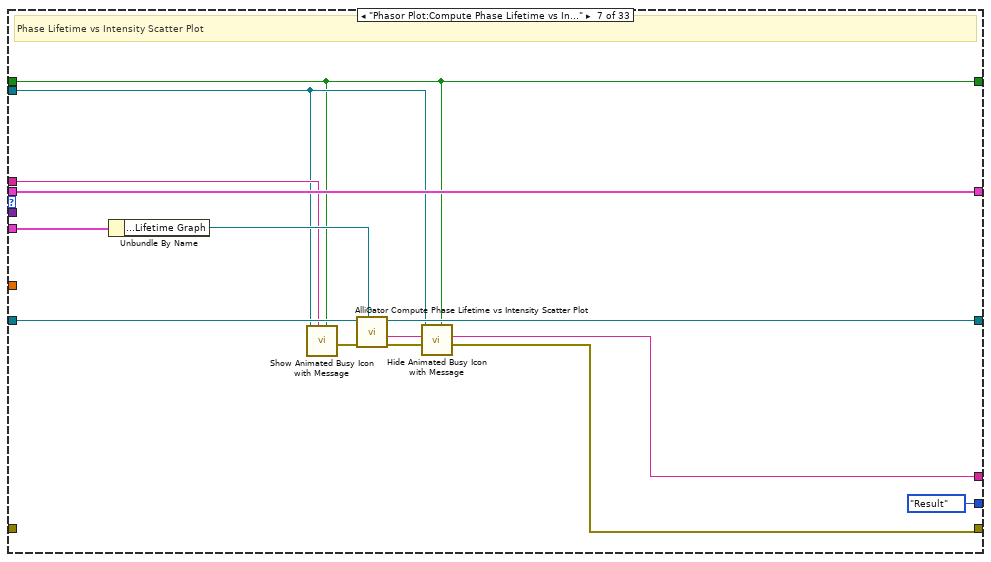
[diagram p14: hidden frame]
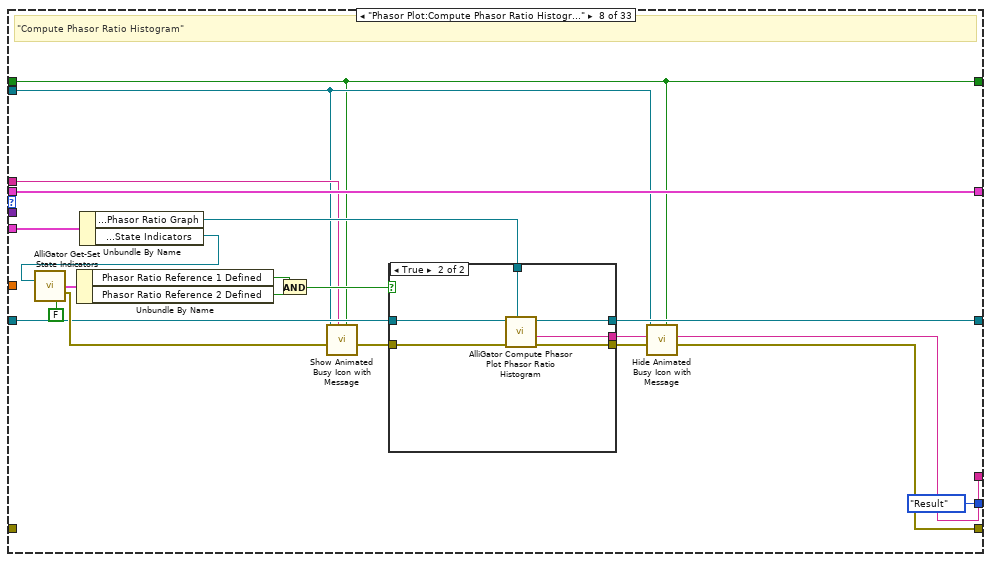
[diagram p15: hidden frame]
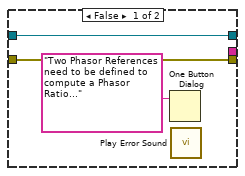
[diagram p16: hidden frame]
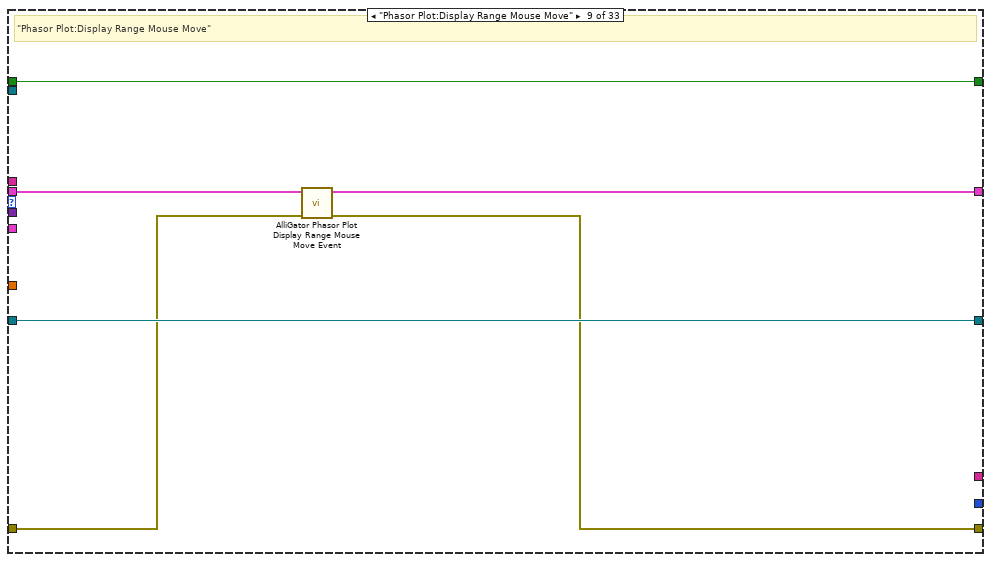
[diagram p17: hidden frame]
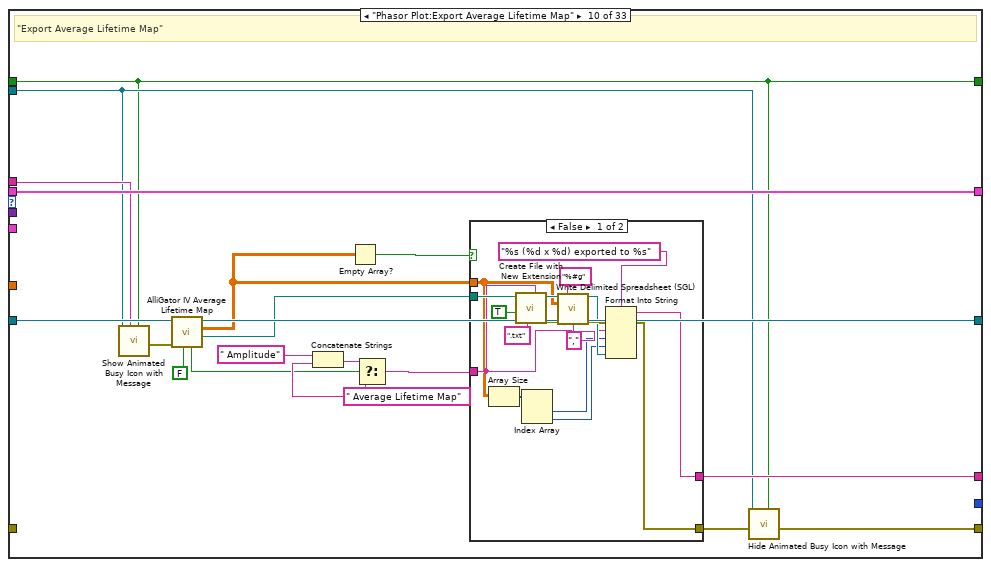
[diagram p18: hidden frame]
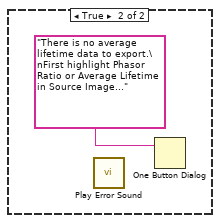
[diagram p19: hidden frame]
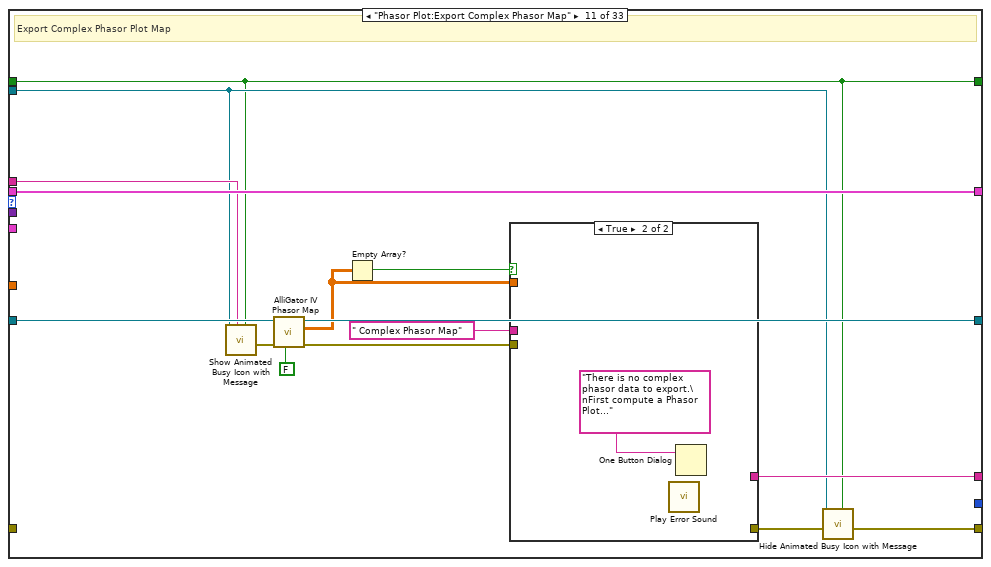
[diagram p20: hidden frame]
diagram:
  # "Author: Xavier Michalet\nCopyright 2025 REGENTS OF THE UNIVERSITY OF CALIFORNIA\n\nRedistribution and use in source and binary forms, with or without modification, are permitted provided that the following conditions are met:\n\n1. Redistributions of source code must retain the above copyright notice, this list of conditions and the following disclaimer.\n\n2. Redistributions in binary form must reproduce the above copyright notice, this list of conditions and the following disclaimer in the documentation and/or other materials provided with the distribution.\n\n3. Neither the name of the copyright holder nor the names of its contributors may be used to endorse or promote products derived from this software without specific prior written permission.\n\nTHIS SOFTWARE IS PROVIDED BY THE COPYRIGHT HOLDERS AND CONTRIBUTORS “AS IS” AND ANY EXPRESS OR IMPLIED WARRANTIES, INCLUDING, BUT NOT LIMITED TO, THE IMPLIED WARRANTIES OF MERCHANTABILITY AND FITNESS FOR A PARTICULAR PURPOSE ARE DISCLAIMED. IN NO EVENT SHALL THE COPYRIGHT HOLDER OR CONTRIBUTORS BE LIABLE FOR ANY DIRECT, INDIRECT, INCIDENTAL, SPECIAL, EXEMPLARY, OR CONSEQUENTIAL DAMAGES (INCLUDING, BUT NOT LIMITED TO, PROCUREMENT OF SUBSTITUTE GOODS OR SERVICES; LOSS OF USE, DATA, OR PROFITS; OR BUSINESS INTERRUPTION) HOWEVER CAUSED AND ON ANY THEORY OF LIABILITY, WHETHER IN CONTRACT, STRICT LIABILITY, OR TORT (INCLUDING NEGLIGENCE OR OTHERWISE) ARISING IN ANY WAY OUT OF THE USE OF THIS SOFTWARE, EVEN IF ADVISED OF THE POSSIBILITY OF SUCH DAMAGE."
  n1 = call "AlliGator Phasor Frequency.vi"() -> ("Phasor Frequency"=w14:dbl[unit])
  n2 = call "AlliGator Event to String.vi"("AlliGator Q Event"="AlliGator Q Event in") -> ("String"=w9:string)  [unwired: 8 in]
  n3 = case shown="\"Phasor Plot:Change Phasor Plot Color Palette\"" "AlliGator Q Event in" {
    selector: "AlliGator Q Event in" -> [_ _ w49 w106 _ _ _ _ _ _ _ _ _ _ _ _ w409 w513 _ _ _ _ _ _ _ _ _ _ _ _ _ _ _]
    tunnel: "Data" -> [_ w34 w48 w107 _ _ _ _ _ _ _ _ _ w380 _ w397 w408 w512 w555 w588 w607 _ w644 w651 w675 _ _ _ w735 _ w765 w782 _]
    tunnel: "AlliGator Q Elements in" -> [w23 w35 w51 w101 w161 w192 w205 w225 w238 w259 w292 w326 w357 w375 w388 w395 w410 w514 w550 w591 w610 w615 w646 w655 w658 w689 w701 w723 w732 w751 w769 w776 w791]
    tunnel: [w23 w35 w50 w101 w160 w192 w205 w225 w237 w259 w292 w326 w356 w374 w388 w394 w404 w508 w550 w591 w610 w615 w646 w655 w658 w688 w700 w723 w731 w748 w768 w775 w791] -> w11
    tunnel: "VI in" -> [_ w30 w47 _ w159 w183 w195 w208 _ w242 w279 w313 w353 _ _ _ w411 w515 w557 _ _ _ w617 _ _ _ w699 _ _ w743 w759 _ _]
    tunnel: w14 -> [_ _ _ _ _ _ _ _ _ _ _ _ _ _ _ _ _ _ _ _ _ _ _ _ _ _ _ _ w726 w745 w761 w773 _]
    tunnel: "Script in" -> [w20 w25 w46 w91 w152 w182 w194 w207 w239 w241 w278 w312 w347 w381 w387 w398 w401 w505 w548 w577 w592 w611 w616 w652 w676 w679 w698 w720 w724 w738 w754 w771 w784]
    tunnel: "error in (no error)" -> [w22 _ _ _ _ _ _ _ w235 _ _ _ _ w372 w383 w396 _ _ w549 _ _ w614 _ w654 w662 _ _ w722 _ _ _ _ _]
    tunnel: [w22 w32 w45 w92 w158 w184 w196 w209 w236 w243 w280 w314 w355 w373 w386 w391 w405 w509 w551 w579 w596 w614 w618 w654 w661 w685 w697 w722 w730 w746 w766 w774 w786] -> w1
    tunnel: "AlliGator Ctrl Refnums" -> [_ w27 w43 w99 w155 w190 w203 w216 _ _ _ _ w352 w377 w385 w390 w407 w511 w554 w581 w604 _ w636 w648 w672 w684 w694 _ _ _ _ _ w789]
    tunnel: "data value reference in" -> [w21 w29 w41 w93 w153 w189 w202 w215 w240 w251 w288 w322 w349 w382 w384 w399 w406 w510 w553 w578 w593 w613 w632 w653 w677 w683 w693 w721 w725 w742 w758 w772 w788]
    tunnel: [w21 w28 w40 w93 w154 w188 w201 w214 w240 w252 w287 w321 w350 w382 w384 w399 w402 w506 w552 w578 w593 w613 w631 w653 w677 w682 w692 w721 w725 w741 w757 w772 w787] -> w19
    tunnel: [_ _ w37 w88 _ w186 w199 w213 _ w246 w283 w317 _ _ _ _ _ w503 _ _ _ _ w625 _ _ _ _ _ _ w739 w755 _ w785] -> w7
    tunnel: w9 -> [_ w24 w38 w83 _ w181 w197 w210 _ w244 w281 w315 w348 _ _ _ w403 w507 w556 _ _ _ w619 _ _ _ w691 _ _ w737 w753 _ _]
    tunnel: [w20 w25 w39 w91 w151 w182 w194 w207 w239 w241 w278 w312 w346 w381 w387 w398 w400 w504 w548 w577 w592 w611 w616 w652 w676 w679 w690 w720 w724 w738 w754 w771 w784] -> w8
    tunnel: [_ _ Text_Format_List."Result" ("Text Format") _ _ Text_Format_List."Result" ("Text Format") Text_Format_List."Result" ("Text Format") Text_Format_List."Result" ("Text Format") _ _ _ _ _ _ _ _ _ Text_Format_List."Result" ("Text Format") _ _ _ _ _ _ _ _ _ _ _ Text_Format_List."Result" ("Text Format") Text_Format_List."Result" ("Text Format") Text_Format_List."Result" ("Text Format") Text_Format_List."Result" ("Text Format")] -> w3
    frame "---- Phasor Plot ----", Default {
      # "\"---- Phaso Plot ----\""
    }
    frame "Phasor Plot:Adjust Phasor Plot Display Range" {
      # "\"Adjust Phasor Plot Display Range\""
      n4 = call-poly "Variant to Data.vi"("Variant"=w34) -> ("Value"=w26:bool)  [unwired: 8 in]
      n5 = call "Show Animated Busy Icon with Message.vi"("Already active? (F)"=w25, "Message"=w24, "Target VI Refnum"=w30) -> ("Error Out"=w31:errorcluster)  [unwired: 8 in]
      n6 = call "AlliGator Adjust Phasor Plot Display Range Wrapper.vi"("error in (no error)"=w31, "Compute Phasor Plot (T)"=w26, "AlliGator Ctrl Refnums"=w27, "Data Value Reference in"=w29) -> ("error out"=w33:errorcluster, "Data Value Reference out"=w28:refnum<data-value>)  [unwired: 6 in]
      n7 = call "Hide Animated Busy Icon with Message.vi"("Already active? (F)"=w25, "Error In"=w33, "Target VI reference"=w30) -> ("Error Out"=w32:errorcluster)  [unwired: 8 in]
    }
    frame "Phasor Plot:Build Phasor Plot" {
      # "\"Build Phasor Plot\""
      n8 = Unbundle By Name(w43) -> ("Phasor Plot Ctrl Refnums.Phasor Plot Active"=w44:refnum<vi>)
      n9 = property class="Bool (strict)"(reference=w44) -> ("Value"=w42:bool)  [unwired: 1 in, 2 out]
      n10 = case shown="True" w42 {
        tunnel: w51 -> [w54 w77]
        tunnel: [w54 w76] -> w50
        tunnel: w49 -> [_ _]
        tunnel: w48 -> [_ w73]
        tunnel: w47 -> [_ w62]
        tunnel: w46 -> [w52 w58]
        tunnel: [_ w59] -> w45
        tunnel: w43 -> [_ w64]
        tunnel: w41 -> [w53 w61]
        tunnel: [w53 w60] -> w40
        tunnel: [w52 w58] -> w39
        tunnel: w38 -> [_ w57]
        tunnel: [_ w55] -> w37
        frame False {
        }
        frame True {
          w56 = FALSE  # This is already called when loading a new Dataset
          n11 = Unbundle By Name(w64) -> ("Registered Events Ctrl Refnums.Phasor Plot Display"=w63:refnum<vi>, "Phasor Plot Ctrl Refnums.Phasor Plot Color Scale"=w66:refnum<vi>, "Registered Events Ctrl Refnums.Phasor Plot Display Range"=w67:refnum<vi>)
          n12 = call-poly "Variant to Data.vi"("Variant"=w73) -> ("String Array"=w69:string[])  [unwired: 8 in]
          n13 = call "AlliGator Get Phasor Plot Display Options.vi"() -> ("error out"=w71:errorcluster, "Phasor Plot Image Elements to Update"=w70:string[])  [unwired: 10 in]
          n14 = Unbundle By Name(w64) -> ("Phasor Plot Ctrl Refnums.Save Phasor Plot"=w65:refnum<vi>)
          n15 = Empty Array?(array=w69) -> (empty?=w72:bool)
          n16 = case shown="True" w56 {
            tunnel: w77 -> [w78 w82]
            tunnel: [w78 w81] -> w76
            frame False {
            }
            frame True {
              n17 = call-poly "AlliGator Add Action(s) to Stack.vi"("Elements Order in Action Stack (Default: 2 BEFORE 1)"=Alligator_Elements_Order_in_Action_Stack."Enqueue 2 BEFORE 1", "Alligator Atomic Action"=T6 {"AlliGator Q Event"=enum."Phasor Plot:Save Phasor Plot Image with Overlay", "Data"=variant}, "Alligator Queue Element 1"=w82) -> ("Alligator Queue Element 1 (+ 2)"=w81:T6[])  [unwired: 7 in, 1 out]
            }
          }
          n18 = Select(t=w70, s=w72, f=w69) -> (s? t:f=w68:string[])
          n19 = call "Show Animated Busy Icon with Message and Abort Button.vi"("Already active? (F)"=w58, "Message"=w57, "Target VI reference"=w62, "Error In"=w71) -> ("Error Out"=w75:errorcluster)  [unwired: 15 in]
          n20 = call "AlliGator Update Phasor Plot Image v2.vi"("Image Control Refnum"=w63, "Phasor Plot Color Scale"=w66, "Error In"=w75, "Phasor Plot Image Elements to Update"=w68, "AlliGator Internal Variables DVR"=w61, "Phasor Plot Display Range Refnum"=w67) -> ("Error Out"=w74:errorcluster, "Message"=w55:string, "AlliGator Internal Variables DVR"=w60:refnum<data-value>)  [unwired: 3 in]
          n21 = call "Hide Animated Busy Icon with Message and Abort Button.vi"("Already active? (F)"=w58, "Target VI reference"=w62, "Error In"=w74) -> ("Error Out"=w59:errorcluster)  [unwired: 16 in]
          n22 = property class="Bool (strict)" props=["Value"](reference=w65) -> ()  [unwired: 1 in, 3 out]
        }
      }
    }
    frame "Phasor Plot:Change Phasor Plot Color Palette" {
      w84 = AlliGator_Variables_List."Phasor Plot:Palette List" ("Alligator Variable")
      # "\"Change Phasor Plot  \""
      n23 = call-poly "Variant to Data.vi"("Variant"=w107) -> ("String"=w105:string)  [unwired: 8 in]
      n24 = call "Alligator Variables Storage.vi"("Get(F)/Set"=FALSE, "AlliGator Variable"=w84) -> ("Data out"=w87:variant)  [unwired: 7 in, 2 out]
      n25 = call-poly "Variant to Data.vi"("Variant"=w87) -> ("String Array"=w86:string[])  [unwired: 8 in]
      n26 = case shown="Default" w105 {
        selector: w105 -> [_ w134 _]
        tunnel: w106 -> [_ _ _]
        tunnel: [w113 w124 w146] -> w104
        tunnel: [w112 w126 w144] -> w103
        tunnel: ["`Palette List Edited" ("Append to Message") w119 _] -> w88
        tunnel: w86 -> [w109 w122 _]
        tunnel: w84 -> [w108 w121 _]
        tunnel: w83 -> [_ w117 _]
        frame "Edit Palette List..." {
          n27 = call "Edit Image Palette List Dialog.vi"("Palette List (in)"=w109) -> ("Palette List (out)"=w116:string[])  [unwired: 10 in]
          n28 = call "Alligator Variables Storage.vi"("Get(F)/Set"=TRUE, "AlliGator Variable"=w108, "Data in"=w116) -> ("Error Out"=w114:errorcluster)  [unwired: 6 in, 2 out]
          n29 = call "AlliGator Check Selected Palette.vi"("Error In"=w114, "Image"=AlliGator_Image_Display_Type."Phasor Plot") -> ("Error Out"=w113:errorcluster, "Image Display Palette Information"=w112:T21)  [unwired: 8 in]
        }
        frame Default {
          n30 = call "Get User Palette Choice.vi"("Palette"=w134) -> ("Error Out"=w129:errorcluster, "Palette Colors"=w132:u32[], "Palette Type"=w133:T22, "Palette Name (# Colors)"=w120:string, "Interpolate?"=w127:bool, "Built-in Palette?"=w125:bool)  [unwired: 3 in, 2 out]
          n31 = Format Into String(format string=": %s", initial string=w117, w120) -> (resulting string=w119:string)  [unwired: 1 in, 1 out]
          n32 = Bundle(cluster=T21 {"Palette Name [# Colors,int?,inv?]"="", "Palette Type"=0, "Palette Colors"=[], "Interpolate?"=FALSE} ("Image Display Palette Information"), "Palette Name [# Colors,int?,inv?]"=w120, "Palette Type"=w133, "Palette Colors"=w132, "Interpolate?"=w127) -> (w126:T21)
          n33 = call "Alligator Variables Storage.vi"("Get(F)/Set"=TRUE, "AlliGator Variable"=AlliGator_Variables_List."Phasor Plot:Palette Information" ("Alligator Variable"), "Error In"=w129, "Data in"=w126) -> ("Error Out"=w123:errorcluster)  [unwired: 5 in, 2 out]
          n34 = case shown="True" w125 {
            tunnel: w123 -> [w142 w143]
            tunnel: [w141 w143] -> w124
            tunnel: w120 -> [w140 _]
            tunnel: w122 -> [w139 _]
            tunnel: w121 -> [w137 _]
            frame False {
              n35 = Build Array (concatenate)(w139, w140) -> (w138:string[])
              n36 = call "Remove Duplicates From 1D Array.vim"("array"=w138) -> ("array with duplicates removed"=w136:string[])  [unwired: 10 in]
              n37 = call "Alligator Variables Storage.vi"("Get(F)/Set"=TRUE, "AlliGator Variable"=w137, "Error In"=w142, "Data in"=w136) -> ("Error Out"=w141:errorcluster)  [unwired: 5 in, 2 out]
            }
            frame True {
            }
          }
        }
        frame "Refresh Image" {
          n38 = call "Alligator Variables Storage.vi"("Get(F)/Set"=FALSE, "AlliGator Variable"=AlliGator_Variables_List."Phasor Plot:Palette Information" ("Alligator Variable")) -> ("Error Out"=w147:errorcluster, "Data out"=w148:variant)  [unwired: 7 in, 1 out]
          n39 = Variant To Data(error in=w147, type=T21 {"Palette Name [# Colors,int?,inv?]"="", "Palette Type"=0, "Palette Colors"=[], "Interpolate?"=FALSE} ("Image Display Palette Information"), Variant=w148) -> (data=w144:T21, error out=w146:errorcluster)
        }
      }
      n40 = Unbundle By Name(w99) -> ("Registered Events Ctrl Refnums.Phasor Plot Display"=w100:refnum<vi>, "Phasor Plot Ctrl Refnums.Phasor Plot Color Scale"=w96:refnum<vi>, "Registered Events Ctrl Refnums.Phasor Plot Display Range"=w98:refnum<vi>)
      n41 = property class="Slide (strict)"(reference=w98) -> (error out=w95:errorcluster, "Value"=w97:cluster{u32, u32})  [unwired: 1 in, 1 out]
      n42 = property class="ColRmp (strict)"(reference=w96, error in=w95) -> (reference out=w94:refnum<vi>, "Scale.High Color"=w89:u32, "Scale.Low Color"=w90:u32)  [unwired: 1 out]
      n43 = call "Image Display Set Color Palette.vi"("Image High Color"=w89, "Image Low Color"=w90, "Error In"=w104, "Image Display Range"=w97, "Image Display Palette Information"=w103, "Display Image Control Refnum"=w100) -> ("Error Out"=w102:errorcluster)  [unwired: 5 in]
      n44 = call "Set Color Ramp Palette v3.vi"("Image High Color"=w89, "Image Low Color"=w90, "error in (no error)"=w102, "Image Display Range"=w97, "Image Display Palette Information"=w103, "ColorRamp in"=w94) -> ("Error Out"=w92:errorcluster)  [unwired: 3 in, 2 out]
    }
    frame "Phasor Plot:Clear Phasor Overlay" {
      # "\"Clear Phasor Overlay\""
      n45 = Unbundle By Name(w155) -> ("Phasor Plot Ctrl Refnums.Phasor Plot Active"=w157:refnum<vi>)
      n46 = property class="Bool (strict)"(reference=w157) -> ("Value"=w156:bool)  [unwired: 1 in, 2 out]
      n47 = case shown="True" w156 {
        tunnel: w161 -> [w164 w174]
        tunnel: [w164 w173] -> w160
        tunnel: w159 -> [_ _]
        tunnel: w152 -> [w162 w165]
        tunnel: [_ w172] -> w158
        tunnel: w155 -> [_ w169]
        tunnel: w153 -> [w163 w167]
        tunnel: [w163 w166] -> w154
        tunnel: [w162 w165] -> w151
        frame False {
        }
        frame True {
          n48 = Unbundle By Name(w169) -> ("Phasor Plot Ctrl Refnums.Save Phasor Plot"=w171:refnum<vi>)
          n49 = Unbundle By Name(w169) -> ("Registered Events Ctrl Refnums.Phasor Plot Display"=w168:refnum<vi>)
          n50 = property class="Bool (strict)"(reference=w171) -> ("Value"=w170:bool)  [unwired: 1 in, 2 out]
          n51 = case shown="True" w170 {
            tunnel: w174 -> [w175 w179]
            tunnel: [w175 w178] -> w173
            frame False {
            }
            frame True {
              n52 = call-poly "AlliGator Add Action(s) to Stack.vi"("Elements Order in Action Stack (Default: 2 BEFORE 1)"=Alligator_Elements_Order_in_Action_Stack."Enqueue 2 BEFORE 1", "Alligator Atomic Action"=T6 {"AlliGator Q Event"=enum."Phasor Plot:Save Phasor Plot Image with Overlay", "Data"=variant}, "Alligator Queue Element 1"=w179) -> ("Alligator Queue Element 1 (+ 2)"=w178:T6[])  [unwired: 7 in, 1 out]
            }
          }
          n53 = call "AlliGator Clear Phasor Image Overlay.vi"("Image Control Refnum"=w168, "AlliGator IV DVR in"=w167) -> ("Error Out"=w172:errorcluster, "AlliGator IV DVR out"=w166:refnum<data-value>)  [unwired: 8 in]
        }
      }
    }
    frame "Phasor Plot:Compute Phase Lifetime Histogram" {
      # "Compute Phase Lifetime Histogram"
      n54 = Unbundle By Name(w190) -> ("Registered Events Ctrl Refnums.Lifetime Graph"=w191:refnum<vi>)
      n55 = call "Show Animated Busy Icon with Message.vi"("Already active? (F)"=w182, "Message"=w181, "Target VI Refnum"=w183) -> ("Error Out"=w185:errorcluster)  [unwired: 8 in]
      n56 = call "AlliGator Compute Phasor Plot Phase Lifetime Histogram.vi"("Lifetime Graph refnum"=w191, "error in (no error)"=w185, "AlliGator IV DVR"=w189) -> ("error out"=w187:errorcluster, "Message"=w186:string, "AlliGator IV DVR"=w188:refnum<data-value>)  [unwired: 6 in]
      n57 = call "Hide Animated Busy Icon with Message.vi"("Already active? (F)"=w182, "Error In"=w187, "Target VI reference"=w183) -> ("Error Out"=w184:errorcluster)  [unwired: 8 in]
    }
    frame "Phasor Plot:Compute Phase Lifetime vs Intensity Scatter Plot" {
      # "Phase Lifetime vs Intensity Scatter Plot"
      n58 = Unbundle By Name(w203) -> ("Registered Events Ctrl Refnums.Lifetime Graph"=w204:refnum<vi>)
      n59 = call "Show Animated Busy Icon with Message.vi"("Already active? (F)"=w194, "Message"=w197, "Target VI Refnum"=w195) -> ("Error Out"=w198:errorcluster)  [unwired: 8 in]
      n60 = call "AlliGator Compute Phase Lifetime vs Intensity Scatter Plot.vi"("Lifetime Graph refnum"=w204, "error in (no error)"=w198, "AlliGator IV DVR"=w202) -> ("error out"=w200:errorcluster, "Message"=w199:string, "AlliGator IV DVR"=w201:refnum<data-value>)  [unwired: 6 in]
      n61 = call "Hide Animated Busy Icon with Message.vi"("Already active? (F)"=w194, "Error In"=w200, "Target VI reference"=w195) -> ("Error Out"=w196:errorcluster)  [unwired: 8 in]
    }
    frame "Phasor Plot:Compute Phasor Ratio Histogram" {
      # "\"Compute Phasor Ratio Histogram\""
      n62 = Unbundle By Name(w216) -> ("Registered Events Ctrl Refnums.Phasor Ratio Graph"=w217:refnum<vi>, "Other AlliGator Ctrl Refnums.State Indicators"=w211:refnum<vi>)
      n63 = call "AlliGator Get-Set State Indicators.vi"("State Indicators Refnum"=w211, "Set (T)/Get"=FALSE) -> ("State Indicator Values"=w222:T32, "Error Out"=w218:errorcluster)  [unwired: 11 in, 1 out]
      n64 = Unbundle By Name(w222) -> ("Phasor Ratio Reference 1 Defined"=w221:bool, "Phasor Ratio Reference 2 Defined"=w220:bool)
      n65 = And(x=w221, y=w220) -> (x .and. y?=w219:bool)
      n66 = call "Show Animated Busy Icon with Message.vi"("Already active? (F)"=w207, "Message"=w210, "Error In"=w218, "Target VI Refnum"=w208) -> ("Error Out"=w212:errorcluster)  [unwired: 7 in]
      n67 = case shown="True" w219 {
        tunnel: [w228 w230] -> w224
        tunnel: w212 -> [w228 w231]
        tunnel: w217 -> [_ w234]
        tunnel: w215 -> [w226 w233]
        tunnel: [w226 w232] -> w214
        tunnel: [_ w229] -> w213
        frame False {
          n68 = One Button Dialog(message="Two Phasor References need to be defined to compute a Phasor Ratio...") -> ()  [unwired: 1 in, 1 out]
          n69 = call "Play Error Sound.vi"() -> ()  [unwired: 27 in, 1 out]
        }
        frame True {
          n70 = call "AlliGator Compute Phasor Plot Phasor Ratio Histogram.vi"("Phasor Ratio Graph refnum"=w234, "error in (no error)"=w231, "AlliGator IV DVR"=w233) -> ("error out"=w230:errorcluster, "Message"=w229:string, "AlliGator IV DVR"=w232:refnum<data-value>)  [unwired: 6 in]
        }
      }
      n71 = call "Hide Animated Busy Icon with Message.vi"("Already active? (F)"=w207, "Error In"=w224, "Target VI reference"=w208) -> ("Error Out"=w209:errorcluster)  [unwired: 8 in]
    }
    frame "Phasor Plot:Display Range Mouse Move" {
      # "\"Phasor Plot:Display Range Mouse Move\""
      n72 = call "AlliGator Phasor Plot Display Range Mouse Move Event.vi"("Error In"=w235, "AlliGator Actions in"=w238) -> ("Error Out"=w236:errorcluster, "AlliGator Actions out"=w237:T6[])  [unwired: 8 in]
    }
    frame "Phasor Plot:Export Average Lifetime Map" {
      w253 = " Average Lifetime Map" ("input 1")
      # "\"Export Average Lifetime Map\""
      n73 = call "Show Animated Busy Icon with Message.vi"("Already active? (F)"=w241, "Message"=w244, "Target VI Refnum"=w242) -> ("Error Out"=w245:errorcluster)  [unwired: 8 in]
      n74 = call "AlliGator IV Average Lifetime Map.vi"("Get (F)/ Set (T)"=FALSE, "error in (no error)"=w245, "AlliGator IV DVR in"=w251) -> ("Single Data Point Path"=w249:path, "[[Average Lifetime]]"=w250:sgl[][], "AlliGator IV DVR out"=w252:refnum<data-value>, "Amplitude Weighted Average Lifeitme"=w248:bool)  [unwired: 4 in, 1 out]
      n75 = Concatenate Strings(" Amplitude" ("input 1"), w253) -> (w254:string)
      n76 = Empty Array?(array=w250) -> (empty?=w257:bool)
      n77 = Select(t=w254, s=w248, f=w253) -> (s? t:f=w256:string)
      n78 = case shown="False" w257 {
        tunnel: [w273 _] -> w258
        tunnel: w249 -> [w271 _]
        tunnel: w250 -> [w263 _]
        tunnel: w256 -> [w266 _]
        tunnel: [w260 _] -> w246
        frame False {
          n79 = Array Size(array=w263) -> (size(s)=w264:i32[])
          n80 = call "Create File with New Extension.vi"("Suffix"=w266, "New File Extension"=".txt" ("New File Extension (with .)"), "Dialog?"=TRUE, "File Path in"=w271) -> ("Error Out"=w269:errorcluster, "New File Path out"=w270:path)  [unwired: 6 in]
          n81 = Index Array(array=w264) -> (element #1=w262:i32, element #2=w261:i32)  [unwired: 2 in]
          n82 = call "Write Delimited Spreadsheet (SGL).vi"("file path (dialog if empty)"=w270, "format (%.3f)"="%#g", "2D data"=w263, "error in (no error)"=w269, "delimiter (\\t)"="," ("delimiter (\\t)")) -> ("new file path (Not A Path if cancelled)"=w272:path, "error out"=w274:errorcluster)  [unwired: 9 in]
          n83 = Format Into String(format string="%s (%d x %d) exported to %s", error in=w274, w266, w262, w261, w272) -> (resulting string=w260:string, error out=w273:errorcluster)  [unwired: 1 in]
        }
        frame True {
          n84 = call "Play Error Sound.vi"() -> ()  [unwired: 27 in, 1 out]
          n85 = One Button Dialog(message="There is no average lifetime data to export.\nFirst highlight Phasor Ratio or Average Lifetime in Source Image...") -> ()  [unwired: 1 in, 1 out]
        }
      }
      n86 = call "Hide Animated Busy Icon with Message.vi"("Already active? (F)"=w241, "Error In"=w258, "Target VI reference"=w242) -> ("Error Out"=w243:errorcluster)  [unwired: 8 in]
    }
    frame "Phasor Plot:Export Complex Phasor Map" {
      # "Export Complex Phasor Plot Map"
      n87 = call "Show Animated Busy Icon with Message.vi"("Already active? (F)"=w278, "Message"=w281, "Target VI Refnum"=w279) -> ("Error Out"=w282:errorcluster)  [unwired: 8 in]
      n88 = call "AlliGator IV Phasor Map.vi"("Get (F)/ Set (T)"=FALSE, "error in (no error)"=w282, "AlliGator IV DVR in"=w288) -> ("error out"=w285:errorcluster, "[[CSG Phasor]]"=w286:csg[][], "AlliGator IV DVR out"=w287:refnum<data-value>)  [unwired: 6 in]
      n89 = Empty Array?(array=w286) -> (empty?=w289:bool)
      n90 = case shown="True" w289 {
        tunnel: [w293 _] -> w291
        tunnel: w286 -> [w301 _]
        tunnel: " Complex Phasor Map" ("input 1") -> [w302 _]
        tunnel: w285 -> [w296 _]
        tunnel: [w294 _] -> w283
        frame False {
          n91 = Array Size(array=w301) -> (size(s)=w298:i32[])
          n92 = call "Create File with New Extension.vi"("Suffix"=w302, "New File Extension"=".txt" ("New File Extension (with .)"), "Error In"=w296, "Dialog?"=TRUE, "File Path in"=path "") -> ("Error Out"=w305:errorcluster, "New File Path out"=w306:path)  [unwired: 5 in]
          n93 = Index Array(array=w298) -> (element #1=w300:i32, element #2=w299:i32)  [unwired: 2 in]
          n94 = call "Files Write Delimited Spreadsheet (CSL).vi"("file path (dialog if empty)"=w306, "format (%.3f)"="%#g", "2D data"=w301, "error in (no error)"=w305, "delimiter (\\t)"="," ("delimiter (\\t)")) -> ("new file path (Not A Path if cancelled)"=w307:path, "error out"=w308:errorcluster)  [unwired: 9 in]
          n95 = Format Into String(format string="%s (%d x %d) exported to %s", error in=w308, w302, w300, w299, w307) -> (resulting string=w294:string, error out=w293:errorcluster)  [unwired: 1 in]
        }
        frame True {
          n96 = call "Play Error Sound.vi"() -> ()  [unwired: 27 in, 1 out]
          n97 = One Button Dialog(message="There is no complex phasor data to export.\nFirst compute a Phasor Plot...") -> ()  [unwired: 1 in, 1 out]
        }
      }
      n98 = call "Hide Animated Busy Icon with Message.vi"("Already active? (F)"=w278, "Error In"=w291, "Target VI reference"=w279) -> ("Error Out"=w280:errorcluster)  [unwired: 8 in]
    }
    frame "Phasor Plot:Export Phasor Ratio Map" {
      # "\"Export Phasor Ratio Map\""
      n99 = call "Show Animated Busy Icon with Message.vi"("Already active? (F)"=w312, "Message"=w315, "Target VI Refnum"=w313) -> ("Error Out"=w316:errorcluster)  [unwired: 8 in]
      n100 = call "AlliGator IV Phasor Ratio Map.vi"("Get (F)/ Set (T)"=FALSE, "error in (no error)"=w316, "AlliGator IV DVR in"=w322) -> ("error out"=w319:errorcluster, "[[Phasor Ratio]]"=w320:sgl[][], "AlliGator IV DVR out"=w321:refnum<data-value>)  [unwired: 6 in]
      n101 = Empty Array?(array=w320) -> (empty?=w323:bool)
      n102 = case shown="True" w323 {
        tunnel: [w341 _] -> w325
        tunnel: w320 -> [w332 _]
        tunnel: " Phasor Ratio Map" ("input 1") -> [w335 _]
        tunnel: w319 -> [w329 _]
        tunnel: [w327 _] -> w317
        frame False {
          n103 = Array Size(array=w332) -> (size(s)=w333:i32[])
          n104 = call "Create File with New Extension.vi"("Suffix"=w335, "New File Extension"=".txt" ("New File Extension (with .)"), "Error In"=w329, "Dialog?"=TRUE, "File Path in"=path "") -> ("Error Out"=w338:errorcluster, "New File Path out"=w339:path)  [unwired: 5 in]
          n105 = Index Array(array=w333) -> (element #1=w331:i32, element #2=w330:i32)  [unwired: 2 in]
          n106 = call "Write Delimited Spreadsheet (SGL).vi"("file path (dialog if empty)"=w339, "format (%.3f)"="%#g", "2D data"=w332, "error in (no error)"=w338, "delimiter (\\t)"="," ("delimiter (\\t)")) -> ("new file path (Not A Path if cancelled)"=w340:path, "error out"=w342:errorcluster)  [unwired: 9 in]
          n107 = Format Into String(format string="%s (%d x %d) exported to %s", error in=w342, w335, w331, w330, w340) -> (resulting string=w327:string, error out=w341:errorcluster)  [unwired: 1 in]
        }
        frame True {
          n108 = call "Play Error Sound.vi"() -> ()  [unwired: 27 in, 1 out]
          n109 = One Button Dialog(message="There is no phasor ratio data to export.\nFirst highlight Phasor Ratio or Average Lifetime in Source Image...") -> ()  [unwired: 1 in, 1 out]
        }
      }
      n110 = call "Hide Animated Busy Icon with Message.vi"("Already active? (F)"=w312, "Error In"=w325, "Target VI reference"=w313) -> ("Error Out"=w314:errorcluster)  [unwired: 8 in]
    }
    frame "Phasor Plot:Highlight Image ROI in Phasor Plot" {
      # "\"Highlight Image ROI in Phasor Plot\""
      n111 = Unbundle By Name(w352) -> ("Phasor Plot Ctrl Refnums.Phasor Plot Active"=w354:refnum<vi>)
      n112 = property class="Bool (strict)"(reference=w354) -> ("Value"=w351:bool)  [unwired: 1 in, 2 out]
      n113 = case shown="True" w351 {
        tunnel: w357 -> [w360 w370]
        tunnel: [w360 w370] -> w356
        tunnel: [_ w367] -> w355
        tunnel: w347 -> [w358 w361]
        tunnel: w352 -> [_ w365]
        tunnel: w353 -> [_ w366]
        tunnel: w349 -> [w359 w364]
        tunnel: [w359 w363] -> w350
        tunnel: w348 -> [_ w362]
        tunnel: [w358 w361] -> w346
        frame False {
        }
        frame True {
          n114 = call "Show Animated Busy Icon with Message.vi"("Already active? (F)"=w361, "Message"=w362, "Target VI Refnum"=w366) -> ("Error Out"=w369:errorcluster)  [unwired: 8 in]
          n115 = call "AlliGator Highlight Image ROI in Phasor Plot Wrapper.vi"("AlliGator Ctrl Refnums"=w365, "error in (no error)"=w369, "AlliGator IV DVR in"=w364) -> ("error out"=w368:errorcluster, "AlliGator IV DVR out"=w363:refnum<data-value>)  [unwired: 7 in]
          n116 = call "Hide Animated Busy Icon with Message.vi"("Already active? (F)"=w361, "Error In"=w368, "Target VI reference"=w366) -> ("Error Out"=w367:errorcluster)  [unwired: 8 in]
        }
      }
    }
    frame "Phasor Plot:Mouse Move" {
      # "\"Phasor Plot:Cursor Move\""
      n117 = Unbundle By Name(w377) -> ("Registered Events Ctrl Refnums.Source Image Display"=w371:refnum<vi>, "Phasor Plot Ctrl Refnums"=w376:T10)
      n118 = Variant To Data(error in=w372, Variant=w380) -> (data=w379:T33, error out=w378:errorcluster)  [unwired: 1 in]
      n119 = call "AlliGator Phasor Plot Mouse Move Event.vi"("Source Image Display Refnum"=w371, "Error In"=w378, "Current Phasor Plot Information Indicators"=w376, "Image User Event Data"=w379, "Alligator Queue Elements in"=w375) -> ("Error Out"=w373:errorcluster, "AlliGator Queue Elements out"=w374:T6[])  [unwired: 5 in]
    }
    frame "Phasor Plot:Update True Phasor Plot Value" {
      n120 = call "AlliGator Display True Phasor Plot Value.vi"("AlliGator Ctrl Refnums"=w385, "error in (no error)"=w383) -> ("error out"=w386:errorcluster)  [unwired: 9 in]
    }
    frame "Phasor Plot:Mouse Up" {
      # "\"Phasor Plot:Mouse Up\""
      n121 = Unbundle By Name(w390) -> ("Phasor Plot Ctrl Refnums"=w389:T10)
      n122 = Variant To Data(error in=w396, Variant=w397) -> (data=w393:T34, error out=w392:errorcluster)  [unwired: 1 in]
      n123 = call "AlliGator Phasor Plot Mouse Up Event.vi"("Current Phasor Plot Information Indicators"=w389, "error in (no error)"=w392, "Phasor Plot Mouse Up Event Data"=w393, "AlliGator Actions in"=w395) -> ("error out"=w391:errorcluster, "AlliGator Actions out"=w394:T6[])  [unwired: 6 in]
    }
    frame "Phasor Plot:Overlay Phasor ROI, Ratio or Map in Source Image" {
      # "\"Overlay Phasor ROI, Ratio or Map in Source Image\""
      n124 = Unbundle By Name(w407) -> ("Phasor Plot Ctrl Refnums.Phasor Plot Active"=w413:refnum<vi>)
      n125 = property class="Bool (strict)"(reference=w413) -> ("Value"=w412:bool)  [unwired: 1 in, 2 out]
      n126 = case shown="True" w412 {
        tunnel: w410 -> [w416 w435]
        tunnel: [w416 w435] -> w404
        tunnel: w409 -> [_ _]
        tunnel: w411 -> [_ w426]
        tunnel: w401 -> [w414 w417]
        tunnel: [_ w434] -> w405
        tunnel: w403 -> [_ w431]
        tunnel: w407 -> [_ w430]
        tunnel: w408 -> [_ w428]
        tunnel: w406 -> [w415 w421]
        tunnel: [w415 w419] -> w402
        tunnel: [w414 w417] -> w400
        frame False {
        }
        frame True {
          n127 = Unbundle By Name(w430) -> ("Dataset Control Refnums.Overlay Mode"=w425:refnum<vi>, "Dataset Control Refnums.Image Color Scale"=w429:refnum<vi>, "Registered Events Ctrl Refnums.Source Image Display"=w433:refnum<vi>, "Registered Events Ctrl Refnums.Phasor Plot Display"=w432:refnum<vi>, "Phasor Plot Ctrl Refnums.Image Overlay Color"=w423:refnum<vi>)
          n128 = property class="Ring (strict)"(reference=w425) -> ("Value"=w424:u16)  [unwired: 1 in, 2 out]
          n129 = property class="ColBox"(reference=w423) -> ("Value"=w422:u32)  [unwired: 1 in, 2 out]
          n130 = call-poly "Variant to Data.vi"("Variant"=w428) -> ("Value"=w427:bool)  [unwired: 8 in]
          n131 = call "Show Animated Busy Icon with Message.vi"("Already active? (F)"=w417, "Message"=w431, "Target VI Refnum"=w426) -> ("Error Out"=w420:errorcluster)  [unwired: 8 in]
          n132 = case shown="0, Default" w424 {
            tunnel: w432 -> [_ w463 _]
            tunnel: w433 -> [w445 w474 w482]
            tunnel: w420 -> [w444 w473 w478]
            tunnel: [w441 w453 w481] -> w418
            tunnel: w421 -> [w450 w470 w480]
            tunnel: [w449 w469 w479] -> w419
            tunnel: w429 -> [w448 w476 w483]
            tunnel: w427 -> [_ w451 _]
            tunnel: w422 -> [_ w462 _]
            frame 2 {
              # "Phasor Color Map"
              n133 = property class="ImageControl"(reference=w445, error in=w444) -> (reference out=w440:refnum<vi>, error out=w437:errorcluster, "Value"=w438:variant)
              n134 = call "Get Color Scale Information.vi"("Error In"=w444, "ColorRamp in"=w448) -> ("Error Out"=w446:errorcluster, "Image Color Scale Information"=w447:T39)  [unwired: 8 in]
              n135 = call-poly "Variant to Data.vi"("Variant"=w438) -> ("Value"=w436:T40)  [unwired: 8 in]
              n136 = Merge Errors(w446, w437) -> (w443:errorcluster)
              n137 = call "AlliGator Overlay Color Map Phasor in Original Image v3.vi"("Image Color Scale Information"=w447, "Error In"=w443, "Source Image Display"=w436, "AlliGator IV DVR in"=w450) -> ("Error Out"=w442:errorcluster, "Source Image Display"=w439:T40, "AlliGator IV DVR out"=w449:refnum<data-value>)  [unwired: 4 in, 1 out]
              n138 = property class="ImageControl"(reference=w440, error in=w442, "Value"=w439) -> (error out=w441:errorcluster)  [unwired: 1 out]
            }
            frame 0, Default {
              # "Phasor ROI"
              n139 = property class="ImageControl"(reference=w463) -> (reference out=w457:refnum<vi>, error out=w454:errorcluster, "Value"=w460:variant, "ROI"=w458:T41)  [unwired: 1 in]
              n140 = property class="ImageControl"(reference=w474, error in=w473) -> (reference out=w471:refnum<vi>, error out=w464:errorcluster, "Value"=w467:variant)
              n141 = call "Get Color Scale Information.vi"("Error In"=w473, "ColorRamp in"=w476) -> ("Error Out"=w475:errorcluster, "Image Color Scale Information"=w468:T39)  [unwired: 8 in]
              n142 = call-poly "Variant to Data.vi"("Variant"=w467) -> ("Value"=w466:T40)  [unwired: 8 in]
              n143 = call-poly "Variant to Data.vi"("Variant"=w460) -> ("Value"=w459:T40)  [unwired: 8 in]
              n144 = Merge Errors(w475, w464, w454) -> (w461:errorcluster)
              n145 = call "AlliGator Highlight Phasor ROI in Original Image v3.vi"("AlliGator IV DVR in"=w470, "Image Color Scale Information"=w468, "Temp Overlay?"=w451, "Source Image Display"=w466, "Phasor Plot Image"=w459, "Phasor Plot ROI"=w458, "Error In"=w461, "Overlay Color"=w462) -> ("AlliGator IV DVR out"=w469:refnum<data-value>, "Source Image Display out"=w465:T40, "Phasor Plot Image Out"=w455:T40, "Error Out"=w456:errorcluster)  [unwired: 3 in, 1 out]
              n146 = property class="ImageControl"(reference=w471, error in=w456, "Value"=w465) -> (error out=w472:errorcluster)  [unwired: 1 out]
              n147 = property class="ImageControl"(reference=w457, error in=w456, "Value"=w455) -> (error out=w452:errorcluster)  [unwired: 1 out]
              n148 = Merge Errors(w472, w452) -> (w453:errorcluster)
            }
            frame 1 {
              # "Phasor Ratio Map"
              n149 = call "AlliGator Get Updated Phasor Ratio References.vi"("error in (no error)"=w478) -> ("error out"=w477:errorcluster)  [unwired: 8 in, 2 out]
              n150 = case shown="No Error" w477 {
                selector: w477 -> [w484 w500]
                tunnel: w483 -> [w498 _]
                tunnel: w482 -> [w496 _]
                tunnel: [w495 w500] -> w481
                tunnel: w480 -> [w493 w501]
                tunnel: [w492 w501] -> w479
                frame No Error {
                  n151 = property class="ImageControl"(reference=w496, error in=w484) -> (reference out=w494:refnum<vi>, error out=w490:errorcluster, "Value"=w491:variant)
                  n152 = call "Get Color Scale Information.vi"("Error In"=w484, "ColorRamp in"=w498) -> ("Error Out"=w497:errorcluster, "Image Color Scale Information"=w485:T39)  [unwired: 8 in]
                  n153 = call-poly "Variant to Data.vi"("Variant"=w491) -> ("Value"=w488:T40)  [unwired: 8 in]
                  n154 = Merge Errors(w497, w490) -> (w489:errorcluster)
                  n155 = call "AlliGator Overlay Phasor Ratio or Derived Quantity on Source Image v3.vi"("Image Color Scale Information"=w485, "Error In"=w489, "Source Image Display"=w488, "AlliGator IV DVR in"=w493) -> ("Error Out"=w486:errorcluster, "Source Image Display out"=w487:T40, "AlliGator IV DVR out"=w492:refnum<data-value>)  [unwired: 4 in, 1 out]
                  n156 = property class="ImageControl"(reference=w494, error in=w486, "Value"=w487) -> (error out=w495:errorcluster)  [unwired: 1 out]
                }
                frame Error {
                  n157 = One Button Dialog(message="Two valid phasor references need to be defined for this analysis...") -> ()  [unwired: 1 in, 1 out]
                }
              }
            }
          }
          n158 = call "Hide Animated Busy Icon with Message.vi"("Already active? (F)"=w417, "Error In"=w418, "Target VI reference"=w426) -> ("Error Out"=w434:errorcluster)  [unwired: 8 in]
        }
      }
    }
    frame "Phasor Plot:Compute Decay of Selected Phasors" {
      # "\"Phasor Plot:Compute Decay of Selected Phasors\""
      n159 = Unbundle By Name(w511) -> ("Phasor Plot Ctrl Refnums.Phasor Plot Active"=w517:refnum<vi>)
      n160 = property class="Bool (strict)"(reference=w517) -> ("Value"=w516:bool)  [unwired: 1 in, 2 out]
      n161 = case shown="True" w516 {
        tunnel: w514 -> [w520 w538]
        tunnel: [w520 w537] -> w508
        tunnel: w513 -> [_ _]
        tunnel: w515 -> [_ w543]
        tunnel: w505 -> [w518 w540]
        tunnel: [_ w547] -> w509
        tunnel: w507 -> [_ w545]
        tunnel: w511 -> [_ w544]
        tunnel: w512 -> [_ _]
        tunnel: w510 -> [w519 w542]
        tunnel: [w519 w541] -> w506
        tunnel: [w518 w540] -> w504
        tunnel: [_ w529] -> w503
        frame False {
        }
        frame True {
          n162 = Unbundle By Name(w544) -> ("Registered Events Ctrl Refnums.Phasor Plot Display"=w546:refnum<vi>)
          n163 = call "Show Animated Busy Icon with Message.vi"("Already active? (F)"=w540, "Message"=w545, "Target VI Refnum"=w543) -> ("Error Out"=w539:errorcluster)  [unwired: 8 in]
          n164 = property class="ImageControl"(reference=w546, error in=w539) -> (error out=w522:errorcluster, "ROI"=w523:T41)  [unwired: 1 out]
          n165 = call "AlliGator Check Current Phasor Image ROI.vi"("Error In"=w522, "ROI Descriptor"=w523) -> ("Error Out"=w521:errorcluster)  [unwired: 7 in, 2 out]
          n166 = call "AlliGator Phasor ROI to Source Image ROI.vi"("Error In"=w521, "Phasor Plot ROI"=w523, "AlliGator IV DVR in"=w542) -> ("Error Out"=w525:errorcluster, "Message"=w529:string, "Source Image ROI"=w530:T25, "AlliGator IV DVR out"=w541:refnum<data-value>)  [unwired: 4 in, 1 out]
          n167 = Bundle By Name(cluster=T24 {"Image Control Label"="Source Image", "ROI Descriptor"={"Global Rectangle"=[], "Contours"=[]}} ("Image ROI"), "ROI Descriptor"=w530) -> (w531:T24)
          n168 = call "AlliGator Settings Storage.vi"("AlliGator Settings List"=AlliGator_Settings_List."Phasor Graph:Phasor Graph Active", "Error In"=w525) -> ("Error Out"=w524:errorcluster, "Variant Data out"=w527:variant)  [unwired: 8 in]
          n169 = call-poly "Variant to Data.vi"("Variant"=w527) -> ("Value"=w526:bool)  [unwired: 8 in]
          n170 = call "AlliGator ROI Analysis Script.vi"("Error In"=w524, "Decay Graph OR Phasor Graph Active?"=w526, "Image ROI"=w531) -> ("Error Out"=w534:errorcluster, "ROI Analysis Script"=w535:T6[])  [unwired: 7 in]
          n171 = call-poly "AlliGator Add Action(s) to Stack.vi"("Elements Order in Action Stack (Default: 2 BEFORE 1)"=Alligator_Elements_Order_in_Action_Stack."Enqueue 2 BEFORE 1", "Error In"=w534, "Alligator Queue Element 2"=w535, "Alligator Queue Element 1"=w538) -> ("Error Out"=w533:errorcluster, "Alligator Queue Element 1 (+ 2)"=w537:T6[])  [unwired: 6 in]
          n172 = call "Hide Animated Busy Icon with Message.vi"("Already active? (F)"=w540, "Error In"=w533, "Target VI reference"=w543) -> ("Error Out"=w547:errorcluster)  [unwired: 8 in]
        }
      }
    }
    frame "Phasor Plot:Phasor at Image Pixel" {
      # "Phasor at Image Pixel"
      n173 = Unbundle By Name(w554) -> ("Phasor Plot Ctrl Refnums"=w563:T10)
      n174 = disable-structure shown="Enabled" {
        disable-tunnel: w555 -> [w571 w576]
        disable-tunnel: [_ w573] -> w568
        disable-tunnel: [w569 w575] -> w567
        disable-tunnel: w549 -> [_ w572]
        frame Disabled {
          n175 = Variant To Data(type=T26 {"Image Control Refnum"=refnum, "Mouse Coordinates"={"Horizontal"=0, "Vertical"=0}} ("Mouse Click Event Data"), Variant=w571) -> (error out=w569:errorcluster)  [unwired: 1 in, 1 out]
        }
        frame Enabled {
          n176 = Variant To Data(error in=w572, type=cluster{"X":i32, "Y":i32} {"X"=0, "Y"=0} ("Last Mouse Position:All Elements"), Variant=w576) -> (data=w573:cluster{"X":i32, "Y":i32}, error out=w575:errorcluster)
        }
      }
      n177 = call "Show Animated Busy Icon with Message.vi"("Already active? (F)"=w548, "Message"=w556, "Error In"=w567, "Target VI Refnum"=w557) -> ("Error Out"=w561:errorcluster)  [unwired: 7 in]
      n178 = call "High Resolution Timing.vi"("Error In"=w561) -> ("elapsed (relative) seconds"=w558:dbl, "Error Out"=w560:errorcluster)  [unwired: 16 in, 1 out]
      n179 = call "AlliGator Get Phasor at Source Image Cursor Location.vi"("error in (no error)"=w560, "AlliGator IV DVR in"=w553, "Mouse Coordinates"=w568) -> ("Error Out"=w562:errorcluster, "Valid Location"=w564:bool, "AlliGator IV DVR out"=w552:refnum<data-value>, "Phasor"=w565:T31)  [unwired: 5 in]
      n180 = call "AlliGator Update Phasor Plot Information at Mouse Location.vi"("Error In"=w562, "Valid?"=w564, "Phasor"=w565, "Current Phasor Plot Information Indicators"=w563) -> ("Error Out"=w566:errorcluster)  [unwired: 6 in, 1 out]
      n181 = call "High Resolution Timing.vi"("relative seconds (NaN)"=w558, "Error In"=w566) -> ("Error Out"=w559:errorcluster)  [unwired: 15 in, 2 out]
      n182 = call "Hide Animated Busy Icon with Message.vi"("Already active? (F)"=w548, "Error In"=w559, "Target VI reference"=w557) -> ("Error Out"=w551:errorcluster)  [unwired: 8 in]
    }
    frame "Phasor Plot:Phasor Plot ROI Selection" {
      # "\"Phasor Plot ROI Selection\""
      n183 = Unbundle By Name(w581) -> ("Registered Events Ctrl Refnums.Phasor Plot Display"=w580:refnum<vi>)
      n184 = Bundle("Action"=AlliGator_ROI_Manager_Actions."Show All ROIs", -1) -> (w585:cluster{"Action":T29, i32})  [unwired: 1 in]
      n185 = Variant To Data(type=w585, Variant=w588) -> (data=w590:cluster{"Action":T29, i32}, error out=w589:errorcluster)  [unwired: 1 in]
      n186 = call "AlliGator Select Phasor Plot ROI.vi"("Error In"=w589, "ROI Selection Data"=w590) -> ("Error Out"=w583:errorcluster, "ROI Descriptor"=w584:T25)  [unwired: 7 in, 1 out]
      n187 = call "Image Display Get-Set ROI.vi"("Get(F)/Set"=TRUE ("Get(F)/Set(T)"), "Error In"=w583, "ROI Descriptor in"=w584, "Image Display Refnum"=w580) -> ("Error Out"=w579:errorcluster)  [unwired: 3 in, 4 out]
    }
    frame "Phasor Plot:Phasor Plot ROI Storage" {
      # "\"Phasor Plot ROI Storage\""
      n188 = Unbundle By Name(w604) -> ("Registered Events Ctrl Refnums.Phasor Plot Display"=w603:refnum<vi>)
      n189 = Variant To Data(type=AlliGator_ROI_Manager_Actions."Show All ROIs" ("Action"), Variant=w607) -> (data=w606:T29, error out=w602:errorcluster)  [unwired: 1 in]
      n190 = call "Image Display Get-Set ROI.vi"("Get(F)/Set"=FALSE ("Get(F)/Set(T)"), "Error In"=w602, "Image Display Refnum"=w603) -> ("Error Out"=w594:errorcluster, "ROI Descriptor out"=w595:T25, "Image Display Refnum (dup)"=w600:T27)  [unwired: 4 in, 2 out]
      n191 = call "ROI to Default ROI Name.vi"("Error In"=w594, "ROI"=w595) -> ("Error Out"=w609:errorcluster, "ROI Type String"=w608:string)  [unwired: 8 in]
      n192 = call-poly "AlliGator Phasor Plot Image ROI Storage [PM].vi"("Error In"=w609, "Current ROI Descriptor"=w595, "Default Name (\"ROI\")"=w608, "Action"=w606) -> ("Error Out"=w597:errorcluster, "Current ROI Descriptor"=w598:T25)  [unwired: 2 in, 4 out]
      n193 = call "Image Display Get-Set ROI.vi"("Get(F)/Set"=TRUE ("Get(F)/Set(T)"), "Error In"=w597, "ROI Descriptor in"=w598, "Image Display Refnum"=w600) -> ("Error Out"=w596:errorcluster)  [unwired: 3 in, 4 out]
    }
    frame "Phasor Plot:Python Function Phasor Plot Event" {
      # "\"Phasor Plot:Python Function Phasor Plot Event\""
      n194 = One Button Dialog(message="Not yet supported....") -> ()  [unwired: 1 in, 1 out]
      n195 = call "Play Error Sound.vi"() -> ()  [unwired: 27 in, 1 out]
    }
    frame "Phasor Plot:Save Phasor Plot Image with Overlay" {
      # "\"Save Phasor Plot Image with Overlay\""
      n196 = call "Show Animated Busy Icon with Message.vi"("Already active? (F)"=w616, "Message"=w619, "Target VI Refnum"=w617) -> ("Error Out"=w620:errorcluster)  [unwired: 8 in]
      n197 = call "AlliGator IV Dataset Path.vi"("Get (F)/ Set (T)"=FALSE, "error in (no error)"=w620, "AlliGator IV DVR in"=w632) -> ("error out"=w626:errorcluster, "[Time-Series Path]"=w629:path[], "Single Data Point Path"=w630:path, "AlliGator IV DVR out"=w631:refnum<data-value>, "Current Dataset"=w628:i32)  [unwired: 4 in]
      n198 = call "AlliGator Get Image File Format.vi"("Error In"=w626) -> ("error out"=w623:errorcluster, "Transparent Mask Color"=w624:u32, "File Extension (.xxx)"=w637:string, "Image File Format"=w638:T42)  [unwired: 7 in]
      n199 = call-poly "Variant to Data.vi"("Variant"=w644) -> ("Value"=w643:bool)  [unwired: 8 in]
      n200 = Unbundle By Name(w636) -> ("Registered Events Ctrl Refnums.Phasor Plot Display"=w645:refnum<vi>)
      n201 = call "AlliGator Get Image Destination File Path.vi"("Image File Extension"=w637, "Image Name Prefix"="Phasor Plot " ("string"), "Error In"=w623, "Current Data Set"=w628, "Time-Series Paths"=w629, "Single Data Point Path"=w630) -> ("Error Out"=w622:errorcluster, "Image File Path"=w642:path)  [unwired: 4 in]
      n202 = call "Image File Dialog (Optional).vi"("Dialog?"=w643, "Error In"=w622, "Image File Format in"=w638, "Default file path in"=w642) -> ("Error Out"=w639:errorcluster, "Image File Format out"=w640:T42, "file path out"=w641:path)  [unwired: 5 in]
      n203 = call "Image Display Save Image.vi"("Mask Color (Transparent)"=w624, "error in (no error)"=w639, "Saved Image File Format"=w640, "File Path in"=w641, "Display Image Control Refnum"=w645) -> ("Error Out"=w634:errorcluster, "File Path out"=w633:path)  [unwired: 5 in]
      n204 = call "Hide Animated Busy Icon with Message.vi"("Already active? (F)"=w616, "Error In"=w634, "Target VI reference"=w617) -> ("Error Out"=w618:errorcluster)  [unwired: 8 in]
      n205 = Format Into String(format string="Phasor plot Image saved with overlay to %s", w633) -> (resulting string=w625:string)  [unwired: 2 in, 1 out]
    }
    frame "Phasor Plot:Set Mouse Move Flag" {
      # "\"Phasor Plot:Set Mouse Move Flag\""
      n206 = call-poly "Variant to Data.vi"("Variant"=w651) -> ("Value"=w650:bool)  [unwired: 8 in]
      n207 = Unbundle By Name(w648) -> ("Registered Events Ctrl Refnums.Phasor Plot Display"=w647:refnum<vi>)
      n208 = call "AlliGator Generic Image Display Mouse Move Flag.vi"("Image Control Refnum"=w647, "Flag (in)"=w650, "Read/Write"=Read-Write."Write") -> ()  [unwired: 6 in, 1 out]
    }
    frame "Phasor Plot:Show Local Phasor Info in Phasor Plot" {
      w670 = 0  # Reference n
      n209 = Unbundle By Name(w672) -> ("Phasor Plot Ctrl Refnums"=w667:T10)
      n210 = Bundle("Current Phasor"=T31 {"g"=nan, "s"=nan}, "Reference n"=w670) -> (w669:cluster{"Current Phasor":T31, "Reference n":i32})  [unwired: 1 in]
      n211 = Variant To Data(error in=w662, type=w669, Variant=w675) -> (data=w674:cluster{"Current Phasor":T31, "Reference n":i32}, error out=w673:errorcluster)
      n212 = Unbundle By Name(w674) -> ("Reference n"=w659:i32, "Current Phasor"=w668:T31)
      n213 = Unbundle By Name(w667) -> ("Reference 1 Button"=w666:refnum<vi>, "Reference 2 Button"=w665:refnum<vi>)
      n214 = call "AlliGator Show Local Phasor Info in Phasor Plot.vi"("error in (no error)"=w673, "Last Mouse Position"=w668, "Current Phasor Plot Information Indicators"=w667) -> ("error out"=w664:errorcluster)  [unwired: 8 in]
      n215 = case shown="2" w659 {
        tunnel: [_ TRUE ("Value")] -> w656
        frame 2 {
        }
        frame 1, Default {
        }
      }
      n216 = Not(x=w656) -> (.not. x?=w657:bool)
      n217 = property class="Bool (strict)"(reference=w665, error in=w664, "Value"=w657, "Visible"=w657) -> (error out=w663:errorcluster)  [unwired: 1 out]
      n218 = property class="Bool (strict)"(reference=w666, error in=w664, "Value"=w656, "Visible"=w656) -> (error out=w660:errorcluster)  [unwired: 1 out]
      n219 = Merge Errors(w660, w663) -> (w661:errorcluster)
    }
    frame "Phasor Plot:Update Phasor Color Map Vertices" {
      # "\"Update Phasor Color Map Vertices\""
      n220 = Unbundle By Name(w684) -> ("Registered Events Ctrl Refnums.Phasor Plot Display"=w681:refnum<vi>)
      n221 = call "AlliGator Update Phasor Color Map Vertices Wrapper.vi"("Image Control Refnum"=w681, "AlliGator IV DVR in"=w683) -> ("error out"=w680:errorcluster, "AlliGator IV DVR out"=w682:refnum<data-value>)  [unwired: 8 in]
      n222 = call-poly "AlliGator Add Action(s) to Stack.vi"("Elements Order in Action Stack (Default: 2 BEFORE 1)"=Alligator_Elements_Order_in_Action_Stack."Enqueue 2 BEFORE 1", "Error In"=w680, "Alligator Atomic Action"=T6 {"AlliGator Q Event"=enum."Phasor Plot:Overlay Phasor ROI, Ratio or Map in Source Image", "Data"=variant}, "Alligator Queue Element 1"=w689) -> ("Error Out"=w685:errorcluster, "Alligator Queue Element 1 (+ 2)"=w688:T6[])  [unwired: 6 in]
    }
    frame "Phasor Plot:Update Phasor Plot Reference" {
      # "\"Update Phasor Plot Reference\""
      n223 = Unbundle By Name(w694) -> ("Phasor Plot Ctrl Refnums.Phasor Plot Active"=w696:refnum<vi>)
      n224 = property class="Bool (strict)"(reference=w696) -> ("Value"=w695:bool)  [unwired: 1 in, 2 out]
      n225 = case shown="True" w695 {
        tunnel: w701 -> [w704 w719]
        tunnel: [w704 w719] -> w700
        tunnel: w699 -> [_ w716]
        tunnel: w698 -> [w702 w710]
        tunnel: [_ w718] -> w697
        tunnel: w694 -> [_ w715]
        tunnel: [w703 w714] -> w692
        tunnel: w693 -> [w703 w713]
        tunnel: w691 -> [_ w711]
        tunnel: [w702 w710] -> w690
        frame False {
        }
        frame True {
          n226 = Unbundle By Name(w715) -> ("Registered Events Ctrl Refnums.Phasor Plot Display"=w712:refnum<vi>)
          n227 = call "Show Animated Busy Icon with Message.vi"("Already active? (F)"=w710, "Message"=w711, "Target VI Refnum"=w716) -> ("Error Out"=w717:errorcluster)  [unwired: 8 in]
          n228 = call "AlliGator Draw Phasor Ratio Reference Overlay Wrapper.vi"("Image Control Refnum"=w712, "error in (no error)"=w717, "Overlay Group"="Phasor Ratio References", "AlliGator IV DVR in"=w713) -> ("error out"=w709:errorcluster, "AlliGator IV DVR out"=w714:refnum<data-value>)  [unwired: 6 in]
          n229 = call "AlliGator Get-Set Phasor Plot Reference is Updated.vi"("Set/Get (F)"=TRUE, "error in (no error)"=w709, "Phasor Plot Reference Updated"=TRUE) -> ("error out"=w708:errorcluster)  [unwired: 7 in, 1 out]
          n230 = call "Hide Animated Busy Icon with Message.vi"("Already active? (F)"=w710, "Error In"=w708, "Target VI reference"=w716) -> ("Error Out"=w718:errorcluster)  [unwired: 8 in]
        }
      }
    }
    frame "Phasor Plot:Update Phasor Plot State" {
      # "UNUSED"
      # "\"Update Phasor Plot State\""
    }
    frame "Phasor Plot:Use Segment Extremities as References" {
      # "\"Use Segment Extremities as References\""
      n231 = Variant To Data(Variant=w735) -> (data=w733:T43[], error out=w734:errorcluster)  [unwired: 2 in]
      n232 = call "AlliGator Use Phasor Plot Segment Extremities as References.vi"("Error In"=w734, "Phasor Frequency"=w726, "Image Points"=w733) -> ("error out"=w727:errorcluster, "Phasor 2"=w728:T31, "Phasor 1"=w729:T31)  [unwired: 6 in]
      n233 = call "AlliGator Update Phasor Ratio References.vi"("Error In"=w727, "Phasor Reference 2"=w728, "Phasor Reference 1"=w729, "AlliGator Q Element in"=w732) -> ("error out"=w730:errorcluster, "Alligator Queue Elements out"=w731:T6[])  [unwired: 6 in]
    }
    frame "Phasor Plot:Use UC/Linear Fit Intersections as References" {
      # "\"Phasor Plot: Use UC/Linear Fit Intersections as References\""
      n234 = call "Show Animated Busy Icon with Message.vi"("Already active? (F)"=w738, "Message"=w737, "Target VI Refnum"=w743) -> ("Error Out"=w744:errorcluster)  [unwired: 8 in]
      n235 = call "AlliGator Use Phasor Plot UC-Linear Fit Intersections as References.vi"("Error In"=w744, "Phasor Frequency"=w745, "AlliGator IV DVR in"=w742) -> ("error out"=w747:errorcluster, "Phasor 2"=w749:T31, "Phasor 1"=w750:T31, "AlliGator IV DVR out"=w741:refnum<data-value>, "Message"=w739:string)  [unwired: 4 in]
      n236 = call "Hide Animated Busy Icon with Message.vi"("Already active? (F)"=w738, "Error In"=w747, "Target VI reference"=w743) -> ("Error Out"=w740:errorcluster)  [unwired: 8 in]
      n237 = call "AlliGator Update Phasor Ratio References.vi"("Error In"=w740, "Phasor Reference 2"=w749, "Phasor Reference 1"=w750, "AlliGator Q Element in"=w751) -> ("error out"=w746:errorcluster, "Alligator Queue Elements out"=w748:T6[])  [unwired: 6 in]
    }
    frame "Phasor Plot:Use UC/Principal Axis Intersections as References" {
      # "\"Use UC/Principal Axis Intersections as References\""
      n238 = call-poly "Variant to Data.vi"("Variant"=w765) -> ("Value"=w762:bool)  [unwired: 8 in]
      n239 = call "Show Animated Busy Icon with Message.vi"("Already active? (F)"=w754, "Message"=w753, "Target VI Refnum"=w759) -> ("Error Out"=w760:errorcluster)  [unwired: 8 in]
      n240 = call "AlliGator Use Phasor Plot UC-Principal Axis Intersections as References.vi"("Phasor Frequency"=w761, "Error In"=w760, "Major Axis?"=w762, "AlliGator IV DVR in"=w758) -> ("error out"=w767:errorcluster, "Phasor 2"=w763:T31, "Phasor 1"=w764:T31, "AlliGator IV DVR out"=w757:refnum<data-value>, "Message"=w755:string)  [unwired: 3 in]
      n241 = call "Hide Animated Busy Icon with Message.vi"("Already active? (F)"=w754, "Error In"=w767, "Target VI reference"=w759) -> ("Error Out"=w756:errorcluster)  [unwired: 8 in]
      n242 = call "AlliGator Update Phasor Ratio References.vi"("Error In"=w756, "Phasor Reference 2"=w763, "Phasor Reference 1"=w764, "AlliGator Q Element in"=w769) -> ("error out"=w766:errorcluster, "Alligator Queue Elements out"=w768:T6[])  [unwired: 6 in]
    }
    frame "Phasor Plot:Use UC/Segment Intersections as References" {
      # "\"Use UC/Segment Intersections as References\""
      n243 = Variant To Data(Variant=w782) -> (data=w780:T43[], error out=w781:errorcluster)  [unwired: 2 in]
      n244 = call "AlliGator Use Phasor Plot UC-Segment Intersections as References.vi"("Error In"=w781, "Phasor Frequency"=w773, "Image Points"=w780) -> ("error out"=w779:errorcluster, "Point 2"=w777:T31, "Point 1"=w778:T31)  [unwired: 6 in]
      n245 = call "AlliGator Update Phasor Ratio References.vi"("Error In"=w779, "Phasor Reference 2"=w777, "Phasor Reference 1"=w778, "AlliGator Q Element in"=w776) -> ("error out"=w774:errorcluster, "Alligator Queue Elements out"=w775:T6[])  [unwired: 6 in]
    }
    frame "Phasor Plot:Weber 2-Component Decomposition" {
      # "2-Component Decomposition"
      n246 = Unbundle By Name(w789) -> ("Registered Events Ctrl Refnums.Lifetime Graph"=w790:refnum<vi>)
      n247 = call "AlliGator Compute Phasor Plot Weber 2-Component Decomposition.vi"("Lifetime Graph refnum"=w790, "AlliGator IV DVR"=w788) -> ("error out"=w786:errorcluster, "Message"=w785:string, "AlliGator IV DVR"=w787:refnum<data-value>)  [unwired: 7 in]
    }
  }
  "Data Value Reference out" <- w19
  "error out" <- w1
  "AlliGator Q Elements out" <- w11
  "Script out" <- w8
  n248 = call "Get Current Message Text Format.vi"("Text Format"=w3) -> ("Error Out"=w2:errorcluster, "Message Formatting"=w6:T2)  [unwired: 8 in]
  n249 = call "AlliGator Package Notebook Messages.vi"("Error In"=w2, "Message Formatting"=w6, "Message"=w7, "AlliGator Q Event in"="AlliGator Q Event in") -> ("[Notebook Message]"=→"[Notebook Message]":T1[])  [unwired: 6 in, 1 out]
